vi "DAQ_PXI_NSCOPE.vi"(0 "Pre-Check Cut-Off (V)":dbl=0.5, 1 "Range Ch0 (A)":dbl=10.0, 2 "Range Ch1 (V)":dbl=10.0, 3 "Frequency (fp)":dbl format="%.10f", 4 "Sample Rate (fs)":dbl format="%#_10g", 5 "# Pre-Checks <1Hz":i32=1, 6 "# Pre-Checks >1Hz":i32=10, 7 "Oscilloscope":refnum<k15>, 8 "FGen Handle":refnum<k15>, 9 "Potentiostat":refnum<visa-resource-name>="Solartron1287", 10 "Auto/Manual \nSignal Averaging":bool, 11 "file path (dialog if empty)":path, 12 "Write Time Data":bool=TRUE, 14 "# Periods (Np)":i32, 16 "# Samples (Ns)":i32, 18 "Manual # Signal Avgs":i32, 20 "Frequency Run #":i32, 21 "Amplitude Run #":i32) -> (15 "Solartron Error":bool, 17 "Error code 1":dbl, 19 "Error code 2":dbl, 22 "Pre-Check Voltage":dbl[](graph), 23 "DAQ Error":errorcluster, 24 "Measurement Complete":bool, 25 "Cut-Off Exceeded":bool, 26 "Avg Data (FFT)":cluster{"f0":dbl, "df":dbl, "magnitude":dbl[]}[](graph), 27 "Avg Data":waveform(dbl)[](graph))   [LabVIEW 2018]
uses:
  <instrlib>/niScope/Controls/niScope trigger slope.ctl
  <instrlib>/niScope/Controls/niScope trigger source digital.ctl
  <instrlib>/niScope/Controls/niScope timestamp type.ctl
  <vilib>/Analysis/baseanly.llb/Mean (DBL).vi
  <instrlib>/niScope/Configure/Trigger/niScope Configure Trigger Digital.vi
  <instrlib>/niScope/Acquire/Fetch/niScope Multi Fetch WDT.vi
  <vilib>/measure/maspectr.llb/FFT Spectrum (Mag-Phase) for 1 Chan.vi
  <vilib>/Waveform/WDTOps.llb/WDT Get Waveform Time Array DBL.vi
  <vilib>/Utility/file.llb/Write To Spreadsheet File (DBL).vi
  <vilib>/measure/NI_MAPro.lvlib
  <vilib>/Analysis/NI_AALBase.lvlib
panel:
  in  "Tab Control 2":enum32{"Time", "Frequency", "Combined I & V"}(tab)
  out "Avg Current":waveform(dbl)(graph)
  out "Avg Voltage":waveform(dbl)(graph)
  out "Raw Current":waveform(dbl)(graph)
  out "Raw Voltage":waveform(dbl)(graph)
  out "Extracted Current":dbl[](graph)
  out "Extracted Voltage":dbl[](graph)
  out "Avg Voltage FFT":cluster{"f0":dbl, "df":dbl, "magnitude":dbl[]}(graph)
  out "Avg Current FFT":cluster{"f0":dbl, "df":dbl, "magnitude":dbl[]}(graph)
  out "Raw Current (FFT)":cluster{"f0":dbl, "df":dbl, "magnitude":dbl[]}(graph)={"f0"=0.0, "df"=0.5129974680086571, "magnitude"=[0.009736686034974913, 0.0068890118193715155, 2.474273316925892e-05, 1.6666181662903927e-05, 0.00018520497481361043, 0.0002020324625728159, 2.9796423917391588e-05, 6.0835799956176654e-05, 3.832061972696404e-05, 8.00163268760432e-05, 6.187686325990989e-05, 0.00010881345143237041, 7.405664232045423e-05, 0.00024529678937191185, 0.00018081723997787064, 0.00013674830034827767, 0.00011578668138923653, 8.132508891103869e-05, 8.436909603493343e-05, 4.3539255195424374e-05, 9.411278296038275e-05, 9.313339616697858e-05, 0.0001904916031194703, 7.18188449372633e-05, 9.515352739845026e-05, 5.8372027209711544e-05, 5.1629081344813335e-05, 0.0001051888984279757, 0.0001017511048336494, 0.00012806290765685684, 0.00023723970211607696, 0.0003284196771042644, 0.00016311109700680552, 7.052872379484058e-05, 6.441909845264623e-05, 8.963484915660137e-05, 4.660091676692494e-05, 1.1473371550415868e-05, 9.8723227863399e-05, 0.00018172145612905383, 0.00036925666576389734, 0.00020825496534972575, 0.00014413683504899518, 0.00011289417085277834, 0.00015953426281898876, 0.00017884377671758568, 8.647602637233157e-05, 3.0610648821725594e-05, 0.0003660063662156784, 0.0005702868602461952, 0.00021324756350599438, 0.00014543243135490178, 0.00014364891510409427, 0.0002982096066457441, 0.0002189892710822117, 7.654008130455015e-05, 9.377522933847826e-05, 0.00018913059395761627, 0.00013606168893038421, 9.838731433003454e-05, 8.098815429925746e-05, 6.508812680274274e-05, 9.860214326190474e-05, 1.1326564628447644e-05, 8.342745136118874e-05, 0.00011200339065280742, 0.00018218423703807567, 6.457659894070577e-05, 5.9605112794137545e-05, 2.0063007064420637e-05, 6.585541984966144e-05, 0.00013007463904747007, 0.00010747989177496173, 6.34156482784896e-05, 3.2140842110284324e-05, 8.656295230172939e-05, 7.554294012686232e-05, 2.9555901488047962e-05, 5.44336799610027e-05, 5.9179056867187395e-05, 3.177348946688188e-05, 0.0001589373764824556, 0.00020007344057657424, 0.00016532419934993018, 0.0002195032937442199, 0.00012792030895095305, 2.6877514530374027e-05, 5.175553268101543e-05, 9.242982765959301e-05, 0.00010891953547865583, 8.794904421914407e-05, 4.997279996143813e-05, 0.00010340449341237465, 0.00017928269490357894, 0.00011400343578560216, 5.16705631906662e-05, 3.995921618814623e-05, 8.877098180368605e-06, 0.00015421538895628968, 0.15339177843082097, 0.3079863886415542, 0.15456404384839195, 0.00012939967441387507, 5.376758334077757e-05, 0.00015723457526394858, 0.00011325594804700243, 0.00010475126580808048, 7.106805692341232e-05, 4.461115944250017e-05, 4.5035497990061865e-05, 0.00014599202683489022, 0.00019381744055934879, 0.00012660788832777155, 0.00010631495550691035, 5.8015657316982975e-05, 4.897213627895938e-05, 3.845893709285947e-05, 4.698686272509827e-05, 5.639004143367423e-05, 0.00013921113063345098, 0.00014851999400272212, 0.00012015584002173139, 2.2919384027760592e-05, 7.072686143507398e-05, 8.646597179868744e-05, 2.3574377975237496e-05, 7.834446303479069e-05, 0.00012318313764416266, 0.00011873834413899145, 7.099237231702384e-05, 2.7940946503255326e-05, 2.6690504994345562e-05, 8.092354678179886e-05, 0.0001481231603102316, 0.00012968992675136646, 3.454139667209186e-05, 6.526155774761239e-05, 9.300479469875524e-05, 3.0392342344455383e-05, 2.6396648157025413e-05, 3.867706349844679e-05, 4.275876334056742e-05, 8.387522147494939e-05, 8.388762532766892e-05, 5.251504295345165e-05, 4.161900465252819e-05, 0.00011192486472668473, 0.000114834446358765, 5.947076800455082e-05, 3.317368982212232e-05, 2.9931490166628703e-05, 2.494336068282783e-05, 8.751156553829414e-05, 7.875126342066757e-05, 8.716511963950046e-05, 7.702867210387553e-05, 2.8050096914227305e-05, 7.303259959720835e-05, 0.00012900223836404033, 7.72471266661751e-05, 1.0825078154982671e-05, 3.588740189973794e-05, 3.412256892415188e-05, 3.374013425044886e-05, 8.078331083064204e-05, 5.692432646868846e-05, 3.3647503843830784e-05, 3.775988882787654e-05, 7.275279727320078e-05, 6.949533452311763e-05, 0.00011832191062124111, 5.60299537837104e-05, 6.523885016889611e-05, 2.414308383480744e-05, 8.488677777026249e-05, 8.059614949570702e-05, 0.00012765831871195473, 0.00015327769066343622, 9.982504766895197e-05, 8.067231055434007e-05, 7.562952469606737e-05, 5.2441647077166705e-05, 8.774798136367469e-05, 8.907484043261529e-05, 4.2626022386031635e-05, 6.629829475941237e-05, 6.007341862699493e-05, 0.00013978145341757655, 0.00011875778781368468, 8.445889428951863e-05, 8.16344140794912e-05, 0.00011652908390162308, 8.686981487586638e-05, 2.0202520212430367e-05, 5.6675358309870864e-05, 6.489700940556412e-05, 3.843468744669687e-05, 8.598439265372556e-05, 5.235259661977289e-05, 1.9505584006020315e-05, 5.4967258789082405e-05, 9.061164932565477e-05, 6.871078242479517e-05, 3.746490793119356e-05, 4.345746570583056e-06, 6.680794809066679e-05, 7.859384577137153e-05, 0.00013946180119439166, 0.00015026973409200598, 0.0001261811098802357, 6.638106768113638e-05, 6.714891135164813e-06, 7.285469936222993e-05, 0.00010025486142062482, 9.340855417396117e-05, 7.13680068546361e-05, 5.4394809470155064e-05, 6.610151345962155e-05, 8.101947070807833e-05, 9.65679717611424e-06, 7.494334931301856e-05, 8.716030749396753e-05, 8.759095241319934e-05, 7.009364663007274e-05, 0.00013040985988452123, 0.00011666946833255358, 8.541439449473249e-05, 7.349157135610967e-05, 5.071127389460994e-05, 9.03494173236385e-05, 0.00013630334293557154, 0.00016550562942030102, 0.00010244158226284989, 0.0005095114593234241, 0.0011040607462522514, 0.0005898797354733062, 8.460699629733707e-05, 6.63279576799476e-05, 7.276767016123001e-05, 9.678912553521579e-05, 0.00011103880036497153, 0.00010390481304795893, 6.723211967444307e-05, 3.3213886943143796e-05, 3.118368973763882e-05, 6.487871614283443e-05, 0.00011403356228342304, 9.961545112336088e-05, 6.042829517827356e-05, 0.0001060634480773622, 6.258637735352707e-05, 1.8767611570095386e-05, 2.2703655562442184e-05, 2.077155298560397e-05, 7.824021568470722e-05, 0.00011626638539470062, 0.00010789538386553134, 6.356140113315058e-05, 2.810239679935883e-05, 4.1775096500033935e-05, 4.607647467623639e-05, 4.235802568480506e-05, 9.104740577434752e-05, 0.00012622488464947946, 0.00011264774436154257, 8.91323109364551e-05, 9.376842798607555e-05, 8.964164862492874e-05, 5.236017496094289e-05, 1.2895474917283831e-05, 5.334432271514443e-05, 8.034685472454221e-05, 0.00011817447952261686, 0.0001016055140793108, 4.093545210834721e-05, 6.397618939265519e-05, 2.7474839384394434e-05, 8.763127512317331e-05, 6.707542704870795e-05, 2.8725232413302552e-05, 1.8017107811668353e-05, 3.8369194145327003e-05, 4.760212941143611e-05, 4.429291876691551e-05, 8.223134513211495e-05, 2.8310310472408665e-05, 4.4706761631630575e-05, 5.816965840260811e-05, 4.35017537930857e-05, 4.467012516597325e-05, 3.946515725898186e-05, 5.691639403547728e-05, 0.00012880744129362161, 9.772451248873228e-05, 3.3912165678514714e-05, 6.17894895191819e-05, 0.00012120627437940271, 0.0001201575820294547, 0.0001085905977033308, 0.00014559566484507596, 8.183886463368417e-05, 2.8953994913944367e-05, 9.657799789209553e-05, 0.00011258550821111594, 4.648209002050687e-05, 5.3750971725136403e-05, 3.245817318073464e-05, 4.9810938136752383e-05, 2.098530153804232e-05, 4.0986434519044244e-05, 1.62171770005793e-06, 6.1003960347686064e-05, 5.709747925701273e-05, 2.741664262162681e-05, 5.508192887786684e-05, 6.104251718802619e-05, 8.362732954581307e-05, 8.839931021231336e-05, 3.189452220701922e-05, 0.00011707895923538106, 0.0001445564751074485, 0.00011442583508313368, 8.905055501835022e-05, 0.00010030213185014967, 0.00010107518845689998, 6.256144387215386e-05, 6.06224533428129e-05, 4.071048604377221e-05, 3.604333177370025e-05, 3.4838493172495606e-05, 5.076623336050464e-05, 8.671222799159577e-05, 0.0001173064723575974, 0.0001490266478294354, 8.565813622945636e-05, 2.993245654881321e-05, 6.189121046054565e-05, 0.00015450812940270522, 0.00016439122756040005, 8.305348425077181e-05, 3.3650880921098876e-05, 5.1460026722577275e-05, 4.4080475501819375e-05, 1.9718762346583145e-05, 4.019192631583561e-05, 6.16280354471133e-05, 4.581307559653348e-05, 7.132076812468776e-05, 7.955624531825839e-05, 4.2853964794850806e-05, 3.6423011063342666e-05, 0.00014801122176452545, 0.00016093044889958237, 0.00010722240371521513, 0.00012350052965298084, 0.00013278815839330737, 0.00012124553101414693, 0.00010594975107531911, 0.00010402056646776084, 6.656200710418502e-05, 5.030208295263895e-05, 0.00013966255877616076, 9.284996782012796e-05, 3.143267597881713e-05, 4.440692708678103e-05, 4.919436029081937e-05, 6.714031688275334e-05, 6.907044421329024e-05, 8.978463840174823e-05, 0.00011999972926478699, 9.624308047471834e-05, 6.685931512769558e-05, 0.0001350330138229978, 7.231584621783556e-05, 0.000124191755290804, 0.00013602537193404393, 5.485262262014689e-05, 3.290832408203692e-05, 8.864254628663135e-05, 9.256403786052085e-05, 0.00010979341528415184, 9.671861892468958e-05, 6.402085877484647e-05, 6.254057256074885e-05, 7.391047540786645e-05, 0.0001375830250966501, 0.00013240222432106118, 7.504311886533425e-05, 4.728428632484807e-05, 4.219163594033604e-05, 4.3894564028540294e-05, 7.402932040891047e-05, 2.0692018869526677e-05, 9.58176723661448e-05, 0.00012859624045696066, 9.468245456234631e-05, 4.58987093578452e-05, 5.973134686001529e-05, 0.00015495789102867437, 0.00015225176035776775, 0.0001152660456485345, 4.3977865615331864e-05, 4.473302645723064e-05, 1.038476669389405e-05, 5.178689049318982e-05, 5.2317526868503626e-05, 7.731241913713737e-05, 4.76983333819832e-05, 5.8764068074275494e-05, 8.050069369254132e-05, 6.607874793802826e-05, 9.048851015371822e-05, 5.0457073148019415e-05, 5.7353792645631936e-05, 8.30515433947444e-05, 2.0042899991487215e-05, 6.113036598742393e-05, 1.946816512274226e-05, 0.00011694111993686107, 7.523172257108798e-05, 9.476294475960118e-05, 0.00013860243809227297, 5.750702760830358e-05, 3.449398233058162e-05, 2.0956641714305812e-05, 2.1504301397232258e-05, 2.7471314957223322e-05, 9.381956771213715e-05, 2.922399583610309e-05, 6.942601588233773e-05, 2.779566295309615e-05, 7.130318946635892e-05, 7.149886430032594e-05, 5.139993358555985e-05, 6.362965788886956e-05, 7.596950087307978e-05, 7.140824565915071e-05, 5.805928359111721e-05, 1.9495487430821023e-05, 4.358710065559153e-05, 9.296638765574948e-05, 5.266407431067206e-05, 7.07958794194355e-05, 8.291348410989419e-05, 6.84661064625638e-05, 7.36777681683598e-05, 8.460517719374566e-05, 5.706680481474532e-05, 5.345143266824526e-05, 4.847036735315841e-05, 2.8214153312565667e-05, 1.578981545533103e-06, 2.420611739278338e-05, 2.5751830567147358e-05, 8.551775498456529e-05, 8.40121859158837e-05, 0.00012635421296699418, 0.00013810496120021876, 9.654466187198543e-05, 7.264826703182078e-05, 8.86819458827062e-05, 3.739617614081658e-05, 2.1572774041456367e-05, 7.405230908668645e-05, 1.0634229827824527e-05, 4.863725308657675e-05, 2.5670242337372567e-05, 0.00030464009896232825, 0.0005215942494986065, 0.00023890089645853916, 5.956385733777223e-05, 3.343738832445387e-05, 7.82343282299264e-05, 7.76107611911919e-05, 3.5356303122637964e-05, 4.9904972391740515e-05, 7.820723201161031e-05, 1.9497081628196724e-06, 9.509232738427502e-05, 0.00012178960632160106, 8.708742033778925e-05, 4.6179588317505504e-05, 7.220912813633792e-05, 9.487815934803574e-05, 0.00013352886336675827, 0.00012944982536255647, 7.347165394621793e-05, 7.378572299473907e-05, 6.868232364642505e-05, 3.152914516619926e-05, 5.081113626186942e-05, 6.410974432711068e-05, 3.3844879974463526e-05, 2.1381637242241187e-05, 8.802911475046838e-05, 7.795492847295635e-05, 4.6401157514948504e-05, 8.296667953849861e-05, 6.300370490185061e-05, 3.9815079382668113e-05, 2.0554859209610595e-05, 2.668634819337046e-05, 3.0594895727724854e-05, 0.00010101228045521858, 7.452174078973984e-05, 7.301396351874438e-05, 5.0361131639115245e-05, 0.00010223885869558667, 7.870120595035575e-05, 3.4195268663717826e-05, 6.993431704109734e-05, 6.784840022167438e-05, 7.877167330164065e-05, 0.00010830351213846695, 4.310256473271412e-05, 5.088589229695461e-05, 3.8889831648106724e-05, 5.313555049798199e-05, 8.937071224748178e-05, 6.366417181000868e-05, 2.6834658547450883e-05, 4.930678366103415e-05, 4.433978719036367e-05, 5.422573682040931e-05, 6.938892015234025e-05, 3.797906339025046e-05, 1.4884417747442926e-05, 2.6187539592185155e-05, 2.2060509314554238e-05, 3.950479262181867e-05, 8.748630975935549e-05, 7.297456341840467e-05, 4.443715821877729e-05, 3.8906913627877566e-05, 8.588731009112597e-05, 0.00011488789170993853, 0.00010509325331548041, 5.8581152791150975e-05, 3.1375583251849565e-05, 0.0001124421149809163, 0.00011647014056875088, 3.698400686923493e-05, 3.932625646119888e-05, 8.815761881254883e-05, 4.9728221439491366e-05, 2.7597546682014243e-05, 4.932919207824848e-05, 6.400269716373524e-05, 4.1488000643268364e-05, 0.00012369789792028514, 8.184587484456742e-05, 2.2257814390089976e-05, 5.836101829959298e-05, 6.053919224290029e-05, 2.160986785547073e-05, 6.684044861256318e-05, 9.936874323743204e-05, 0.00013202011193461338, 0.00014768737320262708, 3.08425032062915e-05, 5.4153579994495385e-05, 1.889707505957545e-05, 4.0234129979895406e-05, 6.708010932003336e-05, 0.0001036576812750676, 1.887118837445916e-05, 4.5727314718384076e-05, 2.1801911253719777e-05, 2.1702554484258357e-05, 6.0057071466645535e-06, 7.726596523730339e-05, 0.00012288780656647378, 0.00010748058602949488, 0.00010927847110088178, 7.566017112974956e-05, 5.434481261853587e-05, 5.2259295868476605e-05, 0.00012236560018837668, 0.00011967397383267307, 0.00013137412972701417, 6.821904344461343e-05, 9.901613754571401e-05, 7.325235838812019e-05, 5.5230935393848205e-05, 0.00011865463490682233, 9.780742744772071e-05, 9.944388518323193e-05, 1.5621224943444166e-05, 5.6737278656342645e-05, 1.130476823449511e-05, 7.567191277607406e-05, 5.661733529281561e-05, 3.697517880681608e-05, 4.7259278007570486e-05, 2.1150705524070954e-05, 5.0408740133679675e-05, 9.742431811289342e-05, 6.043880371443366e-05, 5.4216773363560614e-05, 9.741628508723267e-05, 5.26631847148604e-05, 7.404145166278438e-05, 4.854089759956882e-05, 4.084591046226174e-05, 9.647779744532907e-05, 0.0002086788569078152, 0.0002816364008376485, 0.00012688492199090115, 7.65944894577067e-06, 3.6243190873773735e-05, 5.6219245442062214e-05, 6.482549957968103e-05, 5.952284780214933e-05, 0.00011776869267202251, 6.297764469578426e-05, 5.049489135205378e-05, 8.957388997282253e-05, 0.00012178069093347264, 0.00012994116700553327, 8.65462049613954e-05, 0.00010317293890996919, 8.780074942067528e-05, 3.7070894249722783e-05, 6.063838953162865e-05, 3.8711820408366346e-05, 7.365089012689186e-05, 0.00012167617703242242, 7.463535257145054e-05, 6.744796912337132e-05, 0.00012547238865821364, 7.420593415086781e-05, 1.3265146026887127e-05, 3.778281860584183e-05, 9.263580341779995e-05, 0.00011127482344407767, 5.448048363772164e-05, 9.4835312810856e-05, 0.0001061324583135292, 5.304174882175788e-05, 1.3655344959992683e-05, 7.534164169987058e-05, 0.0001097624891031946, 9.892567197808427e-05, 6.440290146490046e-05, 3.359465023355497e-05, 3.336489617351486e-05, 3.7347271909427096e-05, 1.114351713994515e-05, 1.3280011245846888e-05, 5.7653718644720045e-05, 0.00011376458333905705, 0.00013508519802240597, 0.00015007176037114362, 0.00012605227107725882, 0.00013846080349423415, 9.672450350812372e-05, 8.162393719336778e-05, 8.439681307267638e-05, 4.9305198547823205e-05, 4.916116025882728e-05, 3.679531560280544e-05, 3.381976564598855e-05, 6.800270558935843e-05, 3.883778182696598e-05, 6.619844159553289e-05, 3.61327174348247e-05, 9.899844608661397e-05, 9.641573314022669e-05, 0.00013029877426087654, 9.792622843360607e-05, 9.612773349342937e-06, 0.00010595093656469532, 0.0001062997603506521, 2.0638875230808467e-05, 6.528101510225899e-05, 9.141616308402741e-05, 0.00013000443512000792, 7.352777259967708e-05, 5.8283219779554e-05, 0.00013024724166868325, 7.676376072054004e-05, 4.4004255152320334e-05, 7.377748909308422e-05, 7.282799041503763e-05, 0.00011915254383764491, 0.00013084000234690014, 0.00010875779185399029, 1.8182737075271514e-05, 8.146683382542437e-05, 5.285316001041333e-05, 5.444536450416586e-05, 8.893395805738149e-05, 8.791719908479843e-05, 1.0596102287905125e-05, 5.5376573877938076e-05, 4.445148438988052e-05, 1.3065696408997875e-05, 4.905682607771033e-05, 5.495912985831932e-05, 6.671294454519575e-05, 0.00017614598241608352, 0.00024936876686896593, 0.00023075568028057064, 8.174648183910437e-05, 0.00012832008811656343, 0.00017120686073142003, 8.001791157475066e-05, 5.5262032197503914e-05, 0.00011954837203916514, 0.00014131364608077743, 7.494576556768572e-05, 1.9258150894335585e-05, 2.4689531873113616e-05, 4.100126605219083e-05, 5.5407081228469744e-05, 3.342161763723121e-05, 7.411251564025284e-05, 0.00010266237821433993, 4.365990864847796e-05, 0.00013273480744348552, 0.00010514576472763523, 1.6401965324536744e-05, 3.330547168281681e-05, 5.4876593797890525e-05, 4.1872340037192876e-05, 5.316806803893302e-05, 9.527289462861894e-05, 0.00011932291188269206, 7.07878166763032e-05, 6.140773852560813e-05, 0.00010575849170671164, 3.55693637829357e-05, 0.0001702915367426079, 0.00013198694888416797, 8.719038762157511e-05, 5.8237878386127945e-05, 3.594218835046773e-05, 7.429942605156042e-05, 0.00010349793151274568, 8.551902937563557e-05, 4.514467811784512e-05, 0.00012067802796381594, 7.57907618242714e-05, 7.823011660290687e-05, 0.00010940165977071781, 8.514772365347824e-05, 7.064968219620165e-05, 4.6265666573087246e-05, 3.100548241734962e-05, 4.3039765824007554e-05, 3.557281979382924e-05, 6.790993980024899e-05, 6.976697801962028e-05, 7.416516495684897e-05, 3.066179330092311e-05, 4.82093392389968e-05, 5.6035858550855465e-05, 0.00014238507566795853, 0.00012837569468342303, 4.7836322519587243e-05, 4.090600853776808e-05, 3.8623802708545994e-05, 1.0920860638683462e-05, 4.484421167162386e-05, 4.044967384052889e-05, 5.262324800317312e-05, 6.444345034878788e-05, 0.00012934770560551456, 0.00012532575141136143, 5.113134222634911e-05, 2.5216446871126786e-05, 7.096580006339864e-05, 9.079397535182139e-05, 2.9688993541135436e-05, 0.00012210308543205396, 0.00015444737990201693, 3.5927516997820995e-05, 9.783678721341039e-05, 8.403266144624943e-05, 2.282976613095964e-05, 2.4239904920084537e-05, 2.9592721920004422e-05, 7.465726173416601e-05, 8.068614973947232e-05, 7.093577123693782e-05, 0.00010412829958033035, 9.732216827165277e-05, 5.930575290373523e-05, 0.00011457345386857833, 2.8518905900681316e-05, 2.1936126073443543e-05, 2.8825167081171048e-05, 5.93289117939227e-05, 0.00010209438069501936, 0.0001162370205311875, 4.987420116396371e-05, 0.00011979834313332878, 0.00014711114330424782, 0.000122187845606995, 7.252318340228763e-05, 7.570534940278734e-05, 6.08384890721689e-05, 2.7986426863347572e-05, 4.722924819400313e-05, 5.854346874367302e-05, 9.255160605113158e-05, 0.00010164143314471596, 5.5626096348192946e-05, 2.4038674553347115e-05, 2.8302447295059293e-05, 4.733825719690651e-05, 0.0001127536977895883, 0.00014250397904411297, 0.00010386681879613563, 3.83053126598355e-05, 6.338939647529567e-05, 6.188875910509229e-05, 0.0001299309427061446, 0.0001387621466422242, 0.00010658429185122108, 9.21768261458646e-05, 9.511093033946011e-05, 0.00012935323400315842, 0.00010108674281125153, 3.695887288357596e-05, 2.3353610099248402e-05, 7.621964101659557e-05, 0.0001320341958591496, 0.00010944232875996149, 0.00013403921594062809, 8.008460821005282e-05, 6.328943108465424e-05, 5.2672991184966514e-05, 9.285796299526138e-05, 0.00014128959312560127, 6.506509471810883e-05, 4.2120328583756805e-05, 4.019775672648957e-05, 8.073242584600459e-05, 7.85784793203739e-05, 2.4112589175674725e-05, 4.787838631254602e-05, 1.8493998234257306e-05, 2.102294091265015e-05, 8.585783935453163e-05, 0.00011711203744278809, 0.0001380507068111013, 0.00010905344470843212, 7.628261895217422e-05, 4.667606884598736e-05, 9.718331171415582e-05, 0.00010828985400035679, 4.01628869688618e-05, 9.894226174474573e-05, 4.020560493018181e-05, 1.1689809911468847e-05, 3.0255734845274146e-05, 5.134463794730575e-05, 0.00010907399556691874, 7.973482277266835e-05, 6.722145293054134e-05, 0.0001053169606419433, 4.672146823500862e-05, 5.0539303928871415e-05, 4.8331253016411217e-05, 9.746834923478947e-05, 7.698571800967268e-05, 4.125281773340443e-05, 7.033043184967756e-05, 8.726104290370659e-05, 9.99268254883657e-05, 5.675302645371635e-05, 9.958379275426882e-05, 0.00016827405894896197, 0.00013964759385613767, 8.95549592619375e-05, 7.897571682700118e-05, 6.128746920052035e-05, 6.632258195704656e-05, 6.968881001225131e-05, 7.660022716412855e-05, 0.00010285727745289522, 8.364884815307242e-05, 4.967183102917859e-05, 7.873564670159473e-05, 2.8431073344225065e-05, 0.00011887695069708306, 0.0001386807050420087, 7.845114993305462e-05, 7.501684244765425e-05, 7.655588025221887e-05, 3.417251832136325e-05, 2.465933953351524e-05, 7.675505197378193e-05, 8.774302621367597e-05, 6.954442321748203e-05, 3.4345394042422326e-05, 6.91084206103343e-05, 8.603371623311356e-05, 2.08788859685803e-05, 0.00011747715884471567, 0.0001590319637305697, 9.16542858579216e-05, 4.135831001374284e-05, 4.93906784129331e-05, 6.63191370159788e-05, 7.626841953447927e-05, 5.761164745744449e-05, 5.307108376029597e-05, 5.8823539706247943e-05, 3.441272657484893e-05, 1.297825006753756e-05, 5.789994837285246e-05, 0.00010732593218108915, 7.135371759510655e-06, 0.00010682252977078337, 4.826518290433291e-05, 0.00012217170255594633, 8.898579102329243e-05, 9.04571670529567e-05, 0.000137906168767138, 7.01221516471587e-05, 5.555009661169892e-05, 5.562932049465801e-05, 3.6708423205372413e-05, 3.1710904103314065e-05, 6.77313338328506e-05, 0.00010935049915680121, 7.406214816050558e-05, 3.830638640461101e-06, 8.141981164838396e-05, 9.674105614198826e-05, 3.852252315554934e-06, 5.8673701338300754e-05, 9.560119732944193e-06, 1.2468650315511109e-05, 2.2580391310606328e-05, 8.4699281855885e-05, 3.616555630609264e-05, 6.0242524367222254e-05, 3.7887000817292114e-05, 9.723355489476523e-06, 0.00011497438687740393, 9.887099374371441e-05, 4.968501196928022e-05, 5.030401191366171e-05, 7.697130041308423e-05, 7.913195957848586e-05, 0.0001089804841219723, 0.0001331567938024021, 6.716304425071966e-05, 0.00011416210294702766, 0.00011636997103350444, 5.182024596318364e-05, 5.138795450705537e-05, 2.7076177830046352e-05, 8.565879568166872e-05, 6.0732640651598016e-05, 5.063408706388943e-05, 4.433718014835687e-05, 5.0204412665408934e-05, 4.787562591066475e-05, 6.4906011338989086e-06, 0.00011416805100848756, 0.0001246392522080917, 2.4470860730452252e-05, 6.292790176716217e-05, 5.607839392326423e-05, 6.919123072865869e-06, 4.760260501554702e-05, 6.355851848049534e-05, 5.3553551803857856e-05, 0.00012622125762591353, 7.599771217613932e-05, 5.6808019470107833e-05, 7.239290855550899e-05, 5.849455279273172e-05, 7.934472020911803e-05, 0.00010550105017455192, 5.4620645915706855e-05, 6.86758349387712e-05, 2.8368495390775327e-05, 6.569041242177681e-05, 6.68619356519367e-05, 4.5391570998620266e-05, 2.6026697622941814e-05, 2.9029515552678967e-05, 2.593718695821507e-05, 4.2954470354591866e-05, 3.09612681132032e-05, 4.391713215084827e-05, 4.669939343076136e-05, 5.141138152043193e-05, 3.835081174329836e-05, 1.6017096517240038e-05, 5.39049349126851e-05, 6.465699944047969e-05, 5.210794840750768e-05, 7.468255806654975e-05, 2.3789285868340063e-05, 0.0001184437626939303, 3.443352849048159e-05, 3.578786209871268e-05, 3.547327402633728e-05, 4.3737768060141656e-05, 5.745004643225023e-05, 2.3542254816754582e-06, 5.655420587348942e-05, 8.314204844720425e-05, 5.9657472749715766e-05, 3.664022410474088e-05, 0.0001148120544600091, 8.939767481534439e-05, 5.023100718699245e-05, 0.00010813732941925436, 8.494862157990408e-05, 8.733457168212002e-05, 5.955545570006324e-05, 1.9924278172100827e-05, 7.207335653920181e-05, 5.252879433140767e-05, 5.045635532042773e-05, 8.951432528177735e-05, 1.8460637180872944e-05, 9.222590951048993e-05, 6.954340686450249e-05, 2.1040582881605123e-05, 4.788370106216473e-05, 3.2169955738500416e-05, 9.980405334476289e-05, 4.045951328994319e-05, 8.994470620340262e-05, 0.0001217962045519954, 4.580705365775434e-05, 5.168848122163649e-05, 8.882206357593652e-05, 0.00010217459843757783, 8.487861710537117e-05, 0.00010100790099996582, 0.00013651019546828905, 0.00014885935698358524, 0.00013435973668555912, 0.00012681820332396097, 7.788683493468936e-05, 4.719188328881677e-05, 7.42134396930508e-05, 9.654159845424399e-05, 9.792391262325924e-05, 4.938300479744665e-05, 5.827843733149042e-05, 3.239784247671153e-05, 0.0001651178247974607, 0.00019193477971505418, 0.00021368424717870275, 0.00013185083154650012, 1.9521067740372554e-05, 0.00011647477793580137, 0.00013219511677418103, 4.7091913331635426e-05, 5.592704760289938e-05, 9.229918757236661e-05, 4.045862513745276e-05, 6.129907877749199e-05, 2.5994795835360393e-05, 6.986717008082854e-05, 1.3402979680291646e-05, 3.537934738868749e-05, 0.00010874591203650715, 7.564219759013805e-05, 5.9896174545815454e-05, 6.805640161783559e-05, 2.8185354120430034e-05, 4.027054696526677e-05, 3.4811618518767625e-05, 6.534176687240436e-05, 7.250849374147664e-05, 0.0001555073809743529, 0.0001245114364012905, 8.546002362091024e-05, 0.00012460821285001743, 0.00017201139751436514, 0.00017199255975052118, 7.565527982564014e-05, 7.23877719835643e-05, 0.0001542426407384879, 0.00015573276483068016, 8.94266924162458e-05, 9.082483391685248e-05, 0.00011400344675558218, 1.3158318706717286e-05, 0.00010189119555680978, 6.094548486393501e-05, 6.995790757341798e-05, 9.142914634282154e-05, 5.6710074212175546e-05, 3.5615630698560994e-05, 8.896155900995747e-05, 3.1236595793982005e-05, 7.69757153335617e-05, 6.374685234551762e-05, 3.1149793320846253e-05, 1.4030337410335409e-05, 4.499972918124282e-05, 8.018904215107677e-05, 8.013939385620256e-05, 0.00012356212307987666, 9.661533785137773e-05, 4.400898053700234e-05, 2.1524092202036146e-05, 2.0888608040520335e-05, 2.8210970848255015e-05, 3.52042915785868e-05, 6.470210743827551e-05, 0.00014491759767358054, 0.0001229716959917464, 0.00013064677818916198, 6.944931919737882e-05, 6.2943643625256775e-06, 1.4023829852767115e-05, 2.5367320673109177e-05, 8.793344480173676e-05, 0.00011023073751234149, 8.601579486915851e-05, 7.719475877412213e-05, 9.105332233657286e-05, 6.02837981894214e-05, 2.5261728381191385e-05, 6.323309482102024e-05, 6.600251568271427e-05, 5.469087080920579e-05, 7.1362407823795e-05, 5.603973578987791e-05, 3.0711932252435064e-05, 4.2333118627721086e-05, 6.0543398631587896e-05, 2.503952953985616e-05, 0.00011581570336427287, 9.889701049604456e-05, 4.987980933973253e-05, 1.704673406180222e-05, 2.138043084768542e-05, 3.931841269478685e-05, 4.912854297038053e-05, 6.80522650667397e-05, 0.00011118575599479467, 5.69795060165624e-05, 9.383317094273614e-05, 6.50242539850638e-05, 9.67760844771563e-05, 4.182786376653853e-05, 4.3092827333801965e-05, 6.755793174594356e-06, 8.607607029774266e-06, 5.557776983427308e-05, 0.00010287596735457048, 0.0001159846897373211, 0.00018085811623493077, 0.00011734192003755868, 4.4905187830937135e-05, 6.408202711170145e-05, 0.00011187451004898436, 8.860668065633452e-05, 6.736671323606547e-05, 0.00011029639894262655, 5.3954791360589355e-05, 2.1241782644523725e-05, 1.0381124286379151e-05, 1.9372417418389157e-05, 2.6270507639902297e-05, 7.417575863277701e-05, 0.00016131914111586798, 2.2509271824866267e-05, 0.0001413959480718631, 0.00010788342553119171, 4.897915597212374e-05, 1.6768738982695494e-05, 5.682551383141501e-05, 3.2469246296295584e-05, 2.730718209966202e-05, 4.670975090435728e-05, 5.651485595244382e-05, 6.0553934793525154e-05, 5.209766983284627e-05, 4.116487485013445e-05, 4.022808166339871e-05, 7.598291292934882e-05, 5.346343243672562e-05, 6.210995491712195e-05, 8.230440771696741e-05, 0.00011581622548749921, 9.708832763604018e-05, 9.054211988620269e-05, 0.00010019746047959684, 0.0001000241585182197, 6.0483782737894455e-05, 4.717148726819008e-05, 0.00012416044405786798, 8.501296957991087e-05, 0.00010428848761483963, 0.00015888375923021512, 0.0001592056106987543, 9.219535559178928e-05, 7.262528760170768e-05, 7.117679784352188e-05, 4.27481280885166e-05, 6.064685960260453e-05, 1.1332587355937405e-05, 4.294126765271278e-05, 8.81359432677043e-05, 8.550299799381882e-05, 4.311227336669742e-05, 4.755027850677535e-05, 8.569015674632077e-05, 8.179995549832732e-05, 4.6883847476086586e-05, 4.9330273505091774e-05, 3.037769204953404e-05, 6.871609151127021e-05, 8.536526739843539e-05, 5.396248805577197e-05, 5.1620967281484684e-05, 5.1456862946303014e-05, 4.2652433115283795e-05, 0.0001080544904055672, 7.703919699348674e-05, 1.8221547918931794e-05, 3.0232382465296556e-05, 4.589931518736616e-05, 2.0900031542733726e-05, 6.863004927081564e-05, 0.00017374355797650036, 0.00011652343705188037, 2.1738060754054874e-05, 1.9836622911033635e-05, 2.823543649235006e-05, 7.953501985976011e-05, 7.834497530094624e-05, 0.00012235951285942208, 0.00012843151242013657, 0.00010511024217702175, 5.259322078153344e-05, 4.6286420328241075e-05, 2.88600300106447e-05, 5.891397424689143e-05, 4.8123551507112466e-05, 4.446391483076436e-05, 7.081734855694279e-05, 7.447209064193473e-05, 8.295991090554601e-05, 5.618781898660279e-05, 5.1354457129577643e-05, 9.083447212969017e-05, 6.154890931838974e-05, 4.953098172389299e-05, 4.206468390191532e-05, 9.52545153360766e-05, 0.00013556846728926745, 3.4868557980771985e-05, 8.164743314263412e-05, 5.151548866859173e-05, 9.11155510513629e-05, 6.17406430549882e-05, 8.601213925646853e-05, 0.00013015036634028248, 8.405223491410596e-05, 5.749898498164484e-05, 2.0994360829929272e-05, 5.927473271504225e-05, 9.591805523980466e-05, 3.813789829572376e-05, 0.0001014084740597618, 9.996128195684985e-05, 4.729133626555237e-05, 1.6378855787677934e-05, 6.426790632722436e-05, 8.184663616184083e-05, 0.00010839702687940286, 6.690871343470749e-05, 8.253965986958716e-05, 0.0001246973784528823, 8.747217544938053e-05, 9.636425937037807e-05, 0.00011726190701598256, 3.440639779503234e-05, 0.00013540818941792614, 0.00017054719457821284, 1.5505362529250287e-05, 7.177217805375034e-05, 1.9742007531421337e-05, 5.851138717366113e-05, 0.00013604238423252905, 0.00013683083284163713, 0.00011968899493300909, 7.109103331838126e-05, 5.8856495019582197e-05, 2.796572793047781e-05, 3.085363139621229e-05, 2.81575275507043e-05, 1.388706387496167e-05, 3.051256648284573e-05, 1.3945480049738817e-05, 4.181087351330221e-05, 8.072378899496761e-06, 7.990931711066315e-05, 8.664966942695761e-05, 5.292257837319129e-05, 6.428003834638072e-05, 3.686312542674316e-05, 0.00013453789367506033, 8.391026559501183e-05, 5.7429477640186194e-05, 1.3137523578609169e-05, 2.2945408248717663e-05, 1.7444109217037267e-05, 6.31685176943064e-05, 8.405972046680426e-05, 7.568038590893096e-05, 0.00014789623774038056, 0.00016345173454802633, 5.9143659260903816e-05, 2.355271871607092e-05, 6.50207254924217e-05, 0.0001277433320307822, 8.46824109161955e-06, 0.00010893869330525662, 5.365068338167295e-05, 3.332186339806504e-05, 6.633498511402389e-05, 7.032302427769354e-05, 6.293605649415344e-05, 3.2779160431872945e-05, 5.003840367373862e-05, 8.148365724422335e-05, 9.882527171233261e-05, 5.636912199020016e-05, 3.085180993351448e-05, 5.5244173718013026e-05, 5.502019666713831e-05, 6.505051365827459e-05, 3.9850111141789775e-06, 4.215695342839298e-05, 0.0001060044870478287, 0.0001352374815170716, 1.8998937715323976e-05, 3.5829797254728434e-05, 1.5033253868029578e-05, 5.246643580676588e-05, 0.0001030086140400812, 0.00011147577184680306, 3.642072107283331e-05, 5.726992849962852e-05, 0.0001398177087907839, 0.00014630856414124288, 9.414119181597995e-05, 6.359209645089427e-05, 7.799573345324339e-05, 3.5768659908926674e-06, 0.0001067908834390345, 7.909116601084773e-05, 3.9212939120793605e-05, 6.425301635572063e-05, 7.434819100468811e-05, 3.665951504513878e-05, 1.756992138592397e-05, 5.3833829068806206e-05, 4.4400561838383185e-05, 3.4854072806900566e-05, 5.293535362958484e-05, 2.8980961291710262e-05, 1.0649318805572046e-05, 2.7035756456528955e-05, 3.802596766763527e-05, 7.042548390122817e-05, 6.447321862377597e-05, 1.1445102541184316e-05, 2.4383184836101662e-05, 7.340943785201234e-05, 0.00011455829980455332, 0.00012022826874577315, 0.0001596791046387413, 0.00018775298406475166, 8.420089831255512e-05, 5.0067400228989605e-05, 1.1083266293860374e-05, 1.5552020242010087e-05, 4.653347750589265e-05, 2.3989411178119632e-05, 5.477170338134162e-05, 0.00010014371088002869, 2.2984353404798304e-05, 9.011054525341325e-05, 5.212777210184286e-05, 0.0001355937134226667, 0.00011919918769140552, 8.130366658569784e-05, 3.446692101220835e-05, 0.0001003563947378734, 6.440729547262126e-05, 6.287091225760104e-05, 5.347093032937117e-05, 7.680346774228692e-05, 5.5818744438868304e-05, 3.100357683282677e-05, 1.7242588977592983e-05, 8.135483951968637e-05, 0.0001209829936469434, 0.00011688688534437231, 4.912419526124349e-05, 8.894485008394771e-05, 9.799258821855075e-05, 0.00010807762257419386, 8.729454346275591e-05, 0.00010412181780226692, 6.189699862858598e-05, 3.0235209470920387e-05, 8.253775365930433e-05, 4.1023198533235374e-05, 0.00010472636344886955, 1.0632625210507553e-05, 2.3896957233777144e-05, 3.751791069351541e-05, 8.64452329271966e-05, 0.00010036903007620458, 6.507355385604517e-05, 9.199087509833584e-05, 5.608081582758995e-05, 0.00013121936180527838, 0.000156502862358784, 7.045833505913383e-05, 9.069439608758245e-05, 6.852928326556257e-05, 4.9282801720256094e-05, 6.93913868193009e-05, 4.165715971751554e-05, 0.00012171177514178709, 0.00010146704790968594, 4.906905315422634e-05, 7.965660455216568e-05, 4.906488314702306e-05, 1.024176325587832e-05, 8.399182685138372e-05, 0.00012579142019898774, 4.0100563107338616e-05, 4.9324933631228444e-05, 4.1383990898995025e-05, 7.396270274223919e-05, 8.970708234999438e-05, 8.816364734969336e-05, 0.00012082801087254325, 3.770697363815215e-05, 0.00011826232398438905, 7.229135950909975e-05, 5.336690781724693e-05, 8.354963822375454e-05, 2.3339348912803985e-05, 6.469020497655987e-05, 5.064130096908539e-05, 5.603422529971775e-05, 3.753546116241926e-05, 8.346080175677801e-05, 5.105828421636441e-05, 1.3772559594746388e-05, 1.0500419357342959e-05, 5.836181501549193e-05, 4.429666557845677e-05, 8.463920082676785e-05, 4.084429208069381e-05, 6.148446727108448e-05, 5.829324934446184e-05, 2.9059534594374283e-05, 1.8200181449152194e-05, 2.9013298749062535e-05, 2.1157903229715753e-05, 2.4909756636307545e-05, 5.9396824235009846e-05, 3.4597750875064926e-05, 7.01531323921953e-05, 2.6269865067543734e-05, 0.0001097039032900283, 0.00013097819539911948, 2.637949077043636e-05, 8.136621225148429e-05, 0.00013321592706127047, 9.881237436093312e-05, 3.794107452099959e-05, 1.5434123253124915e-05, 2.071705668804858e-05, 7.854149504225196e-05, 0.00012610977781006094, 0.00010278930531210562, 3.381769885525304e-05, 6.170667723261171e-05, 8.50039144171586e-05, 5.629646286721564e-05, 2.0058513383908546e-05, 5.74526730098044e-05, 7.40415694974769e-05, 7.964952619522259e-05, 4.727187953772571e-05, 9.24774297060932e-05, 0.00010079250907767682, 4.796723482055833e-05, 5.939045811756754e-05, 4.561099444147611e-05, 1.5147435314366943e-05, 1.9479009832401714e-06, 2.5012258712425605e-05, 6.448265791257708e-05, 2.8908738185949957e-05, 2.4829602182734974e-05, 4.209162414483849e-05, 6.622051561880598e-05, 0.00012809633440081158, 0.0001333174764336477, 0.00011519633516021489, 9.199882850616418e-05, 6.718308466116146e-05, 6.619477358073931e-05, 6.24549041101175e-05, 4.6646997281971245e-05, 7.606535665758584e-05, 6.382149608841462e-05, 6.58395326089848e-05, 6.913607587165692e-05, 0.00010314576204833388, 6.392279484441933e-05, 4.658913398904283e-05, 8.619223296222482e-05, 5.344023077991428e-05, 4.1994875998149234e-05, 6.564912168031801e-05, 9.460334353547627e-05, 0.00013307337593759753, 6.070480226900139e-05, 7.42568699635834e-05, 0.0001236092254652738, 5.215927365465155e-05, 5.0805588554635514e-05, 7.596752636148844e-05, 9.597288501832841e-05, 0.00010514543486867016, 0.00010273117411332805, 9.081727998292661e-05, 0.00011445861346242126, 0.00014551786276948577, 0.00015543241010492734, 0.00012032211273871897, 4.055340699527514e-05, 3.39441680160164e-05, 4.021611356129771e-05, 4.846979042047685e-05, 3.528139560736017e-05, 4.4463000731659834e-05, 3.9053083117581076e-05, 3.929185960436038e-05, 4.9628172454793196e-05, 8.204330450857583e-05, 8.944168434142099e-05, 8.691479967161323e-05, 8.082871232078013e-05, 6.0342343549756324e-05, 8.300521466494471e-05, 0.00010945627047477012, 9.114528465499299e-05, 5.9059658886007045e-05, 6.0394959108398155e-05, 8.619000713293784e-05, 9.170073834004933e-05, 7.875930605328551e-05, 0.00010090424100415313, 0.00015638193963645323, 0.00011061037477880064, 6.005192527925918e-05, 7.724630895477524e-05, 3.816941691693574e-05, 2.6777760138001573e-05, 0.00010799217973717106, 7.045983312977735e-05, 1.474584140927438e-05, 3.558795958464629e-05, 4.585423393501645e-05, 8.946001994944166e-05, 0.00011793371738616543, 6.730637563697642e-05, 8.98489806083701e-05, 5.822885149476587e-05, 3.369922165457592e-05, 4.261508552772883e-05, 2.6887192741679545e-05, 4.162386740411925e-05, 3.1168793876430404e-05, 4.597046069679254e-05, 8.7526464824867e-05, 3.6260599806371185e-05, 5.791658915600766e-05, 7.411321117559258e-05, 4.2052907662823005e-05, 5.7062035965089634e-05, 4.363158792611486e-05, 4.7743147444775106e-05, 7.859794288594684e-05, 9.072642886164255e-05, 2.1560854265676325e-05, 5.8735820431875444e-05, 2.5294183114247654e-05, 4.233862839288128e-05, 8.704160734418863e-06, 5.2538890400654945e-05, 8.49857203394752e-05, 4.810969533744059e-05, 4.9423212274192674e-05, 3.301520285289062e-05, 6.20302638228876e-05, 7.322516604443156e-05, 9.317763015494104e-05, 9.109620922760536e-05, 0.00010657134796681009, 7.391588316019145e-05, 1.9653780456160304e-05, 3.687561019767643e-05, 4.50330316455404e-06, 1.4563329932735234e-05, 3.0650720038187365e-05, 0.00011079294905594076, 0.0001231273201769807, 6.0745317595897405e-05, 2.3699432971041623e-05, 1.3163253099269776e-05, 5.200102277736974e-05, 7.166673622716148e-05, 0.00012830849139746665, 0.00014130892061055554, 0.00011004736730139153, 4.758098466601198e-05, 5.7883017839213974e-05, 7.962505514529395e-05, 0.00011167688196843098, 8.794327247697075e-05, 5.8115367223872305e-05, 8.410039975832879e-05, 4.0058700780115186e-05, 6.251684310286954e-05, 0.00011712923299676973, 7.357651725203104e-05, 3.628640510431301e-05, 4.4028895529066666e-05, 6.114377962702075e-05, 9.41284664185419e-05, 8.601390481131111e-05, 7.33695228603279e-05, 0.00010790274521847701, 0.0001072553461176403, 8.942253898758542e-05, 0.00011975275694118204, 0.00016900049442072868, 8.540892650377948e-05, 6.0967074853158266e-05, 3.2900668283086414e-05, 1.761883934805866e-05, 5.791395249878611e-05, 5.8768022283183874e-05, 2.79830111804684e-05, 5.293574040172161e-05, 0.0001315510193344673, 0.0001622739539539606, 0.00010041366770384316, 6.63603960471822e-05, 0.00015747965777463717, 0.00012878560641644074, 7.869153531534173e-05, 3.8059014088214166e-05, 3.769973943621439e-05, 7.742207172954492e-05, 0.00013089412757797647, 8.437661109462401e-05, 2.3324296223741458e-05, 1.0167496017936478e-05, 0.00010029780300179535, 0.00019447555680888684, 0.0001527782270298898, 0.00011884030727830697, 5.937196384587504e-05, 0.00013592129860328509, 0.00011578123354831381, 0.00010345475306570938, 5.50937128004907e-05, 9.704712627245555e-05, 3.3365209177347525e-05, 8.060199359458466e-05, 4.184442707242719e-05, 8.585955431688323e-05, 7.650757949647257e-05, 5.680584546171406e-05, 0.00016185629537601492, 7.9092984220475e-05, 5.510455104733978e-05, 3.54845584077038e-05, 0.00013920058161741384, 0.00013609053638422638, 7.680861189928892e-05, 0.0001687562205747208, 0.00016790589073789464, 9.651391033038544e-05, 4.0192732198884345e-05, 5.247739913211994e-05, 6.164214632583672e-05, 7.233556313460258e-05, 7.176296142846236e-05, 4.236873382092799e-05, 0.00010869221049457684, 0.00012759577785999033, 0.000103702571841759, 6.643467053826662e-05, 3.2770035232537e-05, 4.354708821417443e-05, 5.2289175436611046e-05, 9.783907359228593e-05, 0.00013264098806386033, 8.313405463070077e-05, 5.5194735414876024e-05, 8.692503225526954e-05, 4.756966377211389e-05, 0.00010720466180253656, 6.461366833122605e-05, 4.960281294763827e-05, 7.468503932466735e-05, 3.3496010463612296e-05, 0.00012497113065379812, 0.0001254958924832997, 4.915772645707733e-05, 2.8337615844899863e-05, 5.82863371460653e-05, 9.012194071659063e-05, 0.00012114273428867728, 0.00012446216749867106, 7.496623231657783e-05, 3.696039349454734e-05, 6.761380910193125e-05, 6.254799161472947e-05, 5.462586762783539e-05, 7.329385023661201e-05, 3.313518407250426e-05, 3.6581737132193786e-05, 8.008808689889343e-05, 0.00010710284231672867, 9.328500981498076e-05, 7.555224082660728e-05, 8.323021885733338e-05, 9.279547204802665e-05, 4.0677583586153764e-05, 3.689102450196697e-05, 5.1998453638488155e-05, 6.145274772402466e-05, 9.128816741381892e-05, 6.875827187371332e-05, 9.615302090327267e-05, 0.00011036807115062813, 8.612226657475793e-05, 0.00013531844348037872, 9.843392695596008e-05, 8.622199428216747e-06, 3.8674689645983634e-05, 0.00010630527507886132, 0.00012041630062075119, 6.933143297839332e-05, 5.1904146311599e-05, 7.819505226254796e-05, 2.3294356731909875e-05, 6.22845797345801e-05, 0.00011022691477430783, 5.369604053324257e-05, 5.898245294918871e-05, 7.454244631822826e-05, 7.879306465760291e-05, 0.00011542112111976764, 0.0001255666044061713, 8.777834336422177e-05, 7.215906366287644e-05, 8.285237447945316e-05, 0.00010932001280425939, 0.00011326061020514665, 6.730354951374269e-05, 2.3854805480784416e-05, 3.797582434843099e-05, 0.0001101848432170691, 0.00010909093697863792, 6.820866957751802e-05, 8.58404818202965e-05, 0.0001050570690912771, 7.635888438372816e-05, 2.446602347200826e-05, 5.925245953939786e-05, 5.90862647528598e-05, 5.5661119425029424e-05, 0.00011881461542306238, 0.00013519793202337443, 0.00011144694287596077, 4.487289627654631e-05, 9.39290242668394e-05, 0.0001380918995603799, 0.0001069531367997449, 8.905171488202379e-05, 0.00011936452022966949, 7.075528466570713e-05, 2.92878886815566e-05, 2.1328485908689197e-05, 3.849758796543818e-05, 0.00012075768011660604, 9.658944496122205e-05, 6.398696789497448e-05, 7.320710824906959e-05, 0.00013613994300246026, 9.64148558082593e-05, 4.5229120110167584e-05, 2.994018137707028e-05, 6.48658210872562e-05, 3.009692244233363e-05, 7.491383375523833e-05, 0.0001241587403709238, 0.00010160327357273639, 6.590742095988142e-05, 9.54454814703235e-05, 0.00010831226900531533, 6.421739389598407e-05, 4.994064457500763e-05, 4.136241964313395e-05, 2.616766252396583e-05, 6.66113843813241e-05, 0.00012146425545895542, 0.00010781475109632398, 8.571814066931091e-05, 7.090162024602478e-05, 7.930127910888381e-05, 0.00012961206856157155, 0.00017301280661145287, 7.929453719704741e-05, 9.175365921236214e-06, 3.6644855141514325e-05, 8.31243724371274e-05, 3.4093471591698445e-05, 5.001848398306565e-05, 6.556519425202842e-05, 9.746933013597654e-05, 8.924941232941476e-05, 0.00010870735455352234, 0.00012357968174474653, 0.00011293720755676026, 9.71181336564903e-05, 5.8767772763200484e-05, 2.2683607689607598e-05, 6.500658930637206e-05, 3.237270335970912e-05, 3.03516967301175e-05, 4.1257070322620795e-05, 2.0714862662684896e-05, 5.579677963314373e-05, 0.00011957101263186114, 3.815646663993605e-05, 9.949676788210225e-05, 0.00011348417634772737, 5.789598395396377e-05, 5.636208291119002e-05, 0.00012141526245659619, 0.00012935765334103492, 2.495846196835918e-05, 6.470154347091956e-05, 0.0001218714625828524, 0.0001044306362020955, 3.883853891146619e-05, 7.84091905731201e-05, 0.00010439640342375441, 5.939001056777696e-05, 9.255093128366023e-05, 5.660847225609925e-05, 4.9972528722012964e-05, 8.949477087784792e-05, 8.459018062073713e-05, 5.7738240413584726e-05, 7.92753009390192e-05, 8.313948391090858e-05, 3.104034489963806e-05, 3.4922576519871856e-05, 2.6463805677840565e-05, 6.250103292553367e-05, 5.604349771808582e-05, 1.88850331341025e-05, 5.8078680196711065e-05, 6.984409871092298e-05, 7.95380931768891e-05, 6.807802386435105e-05, 5.9558140436214085e-05, 7.213971585300156e-05, 0.00010742956381038589, 5.608720604574932e-05, 5.297999269479671e-05, 5.636252081641768e-05, 4.2765736927046717e-05, 7.929207579677481e-05, 5.170054352031662e-05, 3.235844291132538e-05, 7.189127482591416e-05, 5.9485339850344885e-05, 2.2872227746178528e-05, 9.034371069921884e-06, 3.370541701959574e-05, 2.0341990707233336e-05, 6.485112257081139e-05, 9.730721318653941e-05, 0.00013873490379153012, 6.815977787487433e-05, 6.730183298348057e-05, 4.0830836888972415e-05, 5.6950738439967104e-06, 3.378526679093192e-05, 5.783801512336395e-05, 0.00011130273912585958, 7.37316408538385e-05, 8.717100093151282e-05, 4.2391260742172246e-05, 9.640844437892159e-05, 0.00010896010978726657, 4.063961127776657e-05, 5.8592322316166396e-05, 9.832190134104383e-05, 7.784131189198688e-05, 7.339203779891448e-05, 8.052290444603476e-05, 5.254474607529348e-05, 1.6934990974464035e-05, 6.473913076511907e-05, 1.2253368037900021e-05, 9.137512258302066e-05, 0.0001121488414027969, 8.571449679469415e-05, 2.6091871960842114e-05, 0.0001303018666404853, 7.20433056337579e-05, 6.249695845606734e-06, 5.489101064908021e-05, 7.039293880441748e-05, 6.844346660738281e-05, 3.243799103428434e-05, 5.122963053040751e-05, 9.277836772132665e-05, 9.663316816260325e-05, 9.047055517785077e-05, 5.313887628073664e-05, 7.291040988571511e-05, 3.123093674094989e-05, 1.6902181789714648e-05, 5.8728408015545155e-05, 3.3124873390271e-05, 2.7698820224219902e-05, 0.00010837994080925189, 0.00014288382367119351, 6.5139745755687e-05, 2.998039199004387e-05, 5.562833455792361e-05, 9.781954934865145e-05, 0.00012007322323158979, 9.328482781678234e-05, 6.240056137756578e-05, 6.58169551672311e-05, 6.12327487763538e-05, 2.817537422284425e-05, 1.7917150359805564e-05, 1.739665383825207e-05, 2.8118451033007985e-06, 2.6522798148353122e-05, 6.631545781670024e-05, 5.165684024618699e-05, 2.1631026538407133e-05, 1.1809912122062645e-06, 3.8807377305429504e-05, 8.913030111518458e-05, 9.70204491874142e-05, 7.412257848450545e-05, 5.8034736074653764e-05, 6.92480484683944e-05, 4.836615311561655e-05, 3.786108395810475e-05, 7.778360935110772e-05, 9.985966569416114e-05, 6.592200902834201e-05, 3.251398386722715e-05, 8.960290062200105e-05, 0.0001342295460552666, 0.0001589347808199238, 0.00012586143570128094, 7.762763233104493e-05, 6.242986028726998e-05, 4.88555914538052e-05, 3.827872144358987e-05, 3.1267453273230836e-05, 1.6626235169223447e-05, 3.828848833350613e-05, 4.694971005164314e-05, 0.000101184054728353, 0.000182784623312052, 0.00016163841824241604, 5.548112411903441e-05, 7.191554604936042e-05, 2.713661483731405e-05, 8.234636339507204e-05, 7.789460847959719e-05, 5.8431089279906395e-05, 0.00010351660014206386, 9.212425351375383e-05, 6.281782578978951e-05, 2.9572266772697958e-05, 0.00011954893594033768, 0.0002466339638049367, 0.00017645789879917187, 8.086077112416246e-05, 0.00011649862570561313, 0.00010676502194584346, 4.379470710757741e-05, 2.992337493656947e-05, 1.707268961008472e-05, 1.093855233850776e-05, 1.728294165919905e-05, 5.3555638739388283e-05, 3.3636160153926004e-05, 2.7048489615121222e-05, 5.552535854710012e-05, 3.5083616718634565e-05, 0.000113775469576003, 7.942127126999557e-05, 3.543442824298634e-05, 5.045362377409201e-05, 0.00016534046136717142, 0.00018311315284389346, 6.429406871878587e-05, 1.732298024604163e-05, 9.352489697415701e-05, 0.00019664270839550476, 0.00018165653164511653, 6.744277337521831e-05, 2.4156228945603937e-05, 7.857838172448876e-05, 9.338578546972164e-05, 7.251833357484212e-05, 4.103191180296767e-05, 4.4601976834397864e-05, 5.581693629735729e-05, 3.509515954301607e-05, 2.2575159437128305e-05, 4.3728589582796625e-05]}
  out "Raw Voltage (FFT)":cluster{"f0":dbl, "df":dbl, "magnitude":dbl[]}(graph)
  out "Raw I & V":waveform(dbl)[](graph)
  in  "Tab Control":enum32{"Inputs", "Status", "Output"}(tab)
  in  "Error In (No Error)":errorcluster
  out "Signal Average #":i32
  out "Mean Current":dbl format="%0.2f"
  out "Mean Voltage":dbl format="%0.2f"
  out "Sample Multiplier":i32
  out "Characters Read":string
  out "Pre-Check Active":bool
  out "Pre-Check Pot Instr Error":errorcluster
  out "dt (DAQ)":dbl
  out "Final Sampling Rate":dbl
  out "Data Size (low freq)":dbl
  out "Data Size":dbl
  out "Pre-Check (Real-Time)":dbl(graph)
  out "wfm info":T1(array[cluster]) caption="NISCOPE wfm info" {"reserved2" format="%.2f"; "reserved1" format="%.2f"; "offset" format="%^.3e"; "gain" format="%^.3e"; "xIncrement" format="%^.3e"; "relativeInitialX" format="%^.3e"; "absoluteInitialX" format="%^.3e"}
  out "Output Data Array":dbl[][](array[numeric])
  # "Raw DAQ Output"
  # "Post Low-Freq Filtering"
  # "Post Signal Averaging"
  # "Raw DAQ Output (FFT)"
  # "Post Signal Averaging"
  # "Sweep Progress"
  # "Sampling Info"
  # "Signal Averaging"
  # "Bias Reject"
  # "Pre-Check"
  # "DAQ Settings"
  # "Write to File"
  # "Sampling Info"
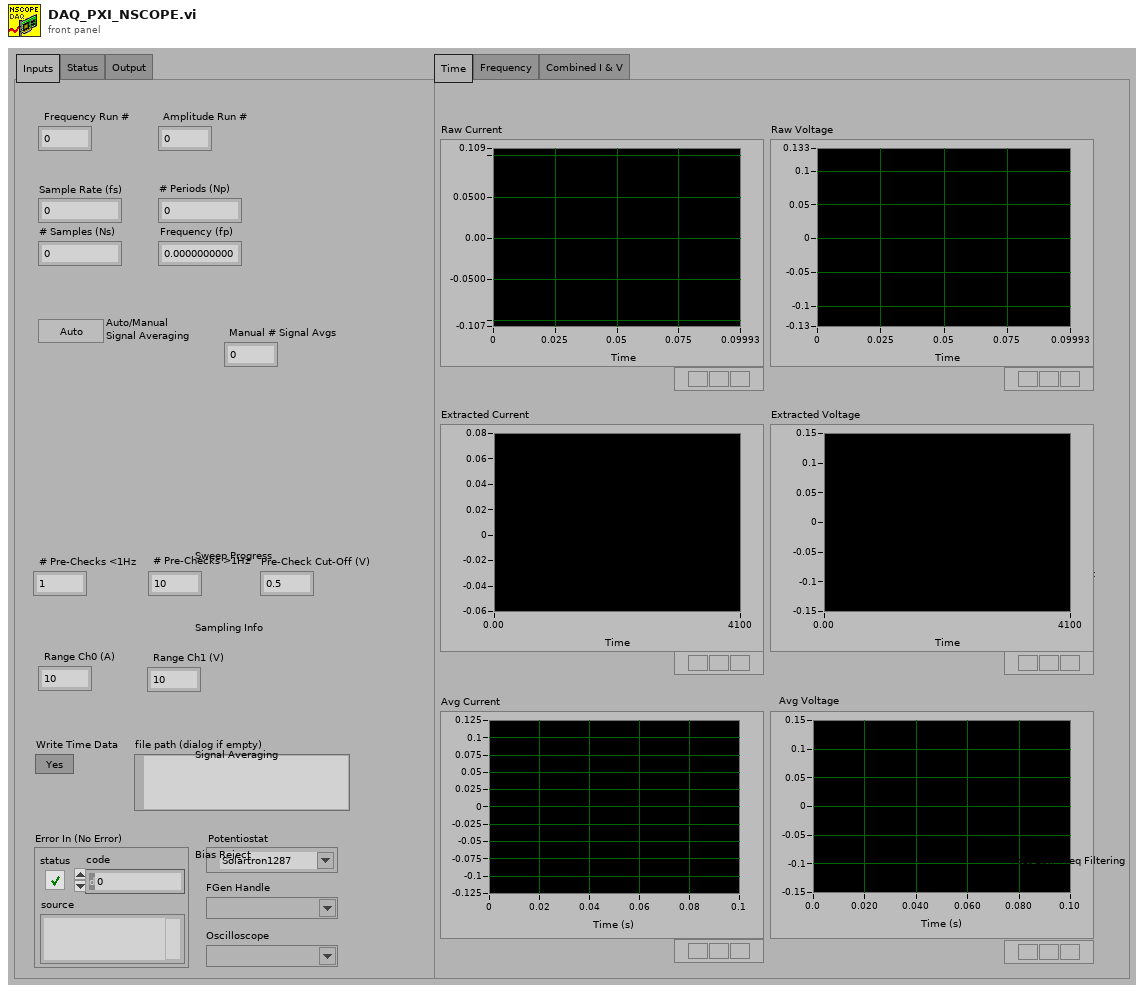
[diagram p1: front panel]
types:
  T1 = cluster{"actualSamples":i32, "absoluteInitialX":dbl, "relativeInitialX":dbl, "xIncrement":dbl, "offset":dbl, "gain":dbl, "reserved1":dbl, "reserved2":dbl}[]
  T2 = typedef "niScope trigger source digital.ctl" = string
  T3 = typedef "niScope timestamp type.ctl" = i32
  T4 = typedef "niScope trigger slope.ctl" = i32
  T5 = enum16{"None ", "Hanning", "Hamming", "Blackman-Harris", "Exact Blackman", "Blackman", "Flat Top", "4 Term B-Harris ", "7 Term B-Harris", "Low Sidelobe"}
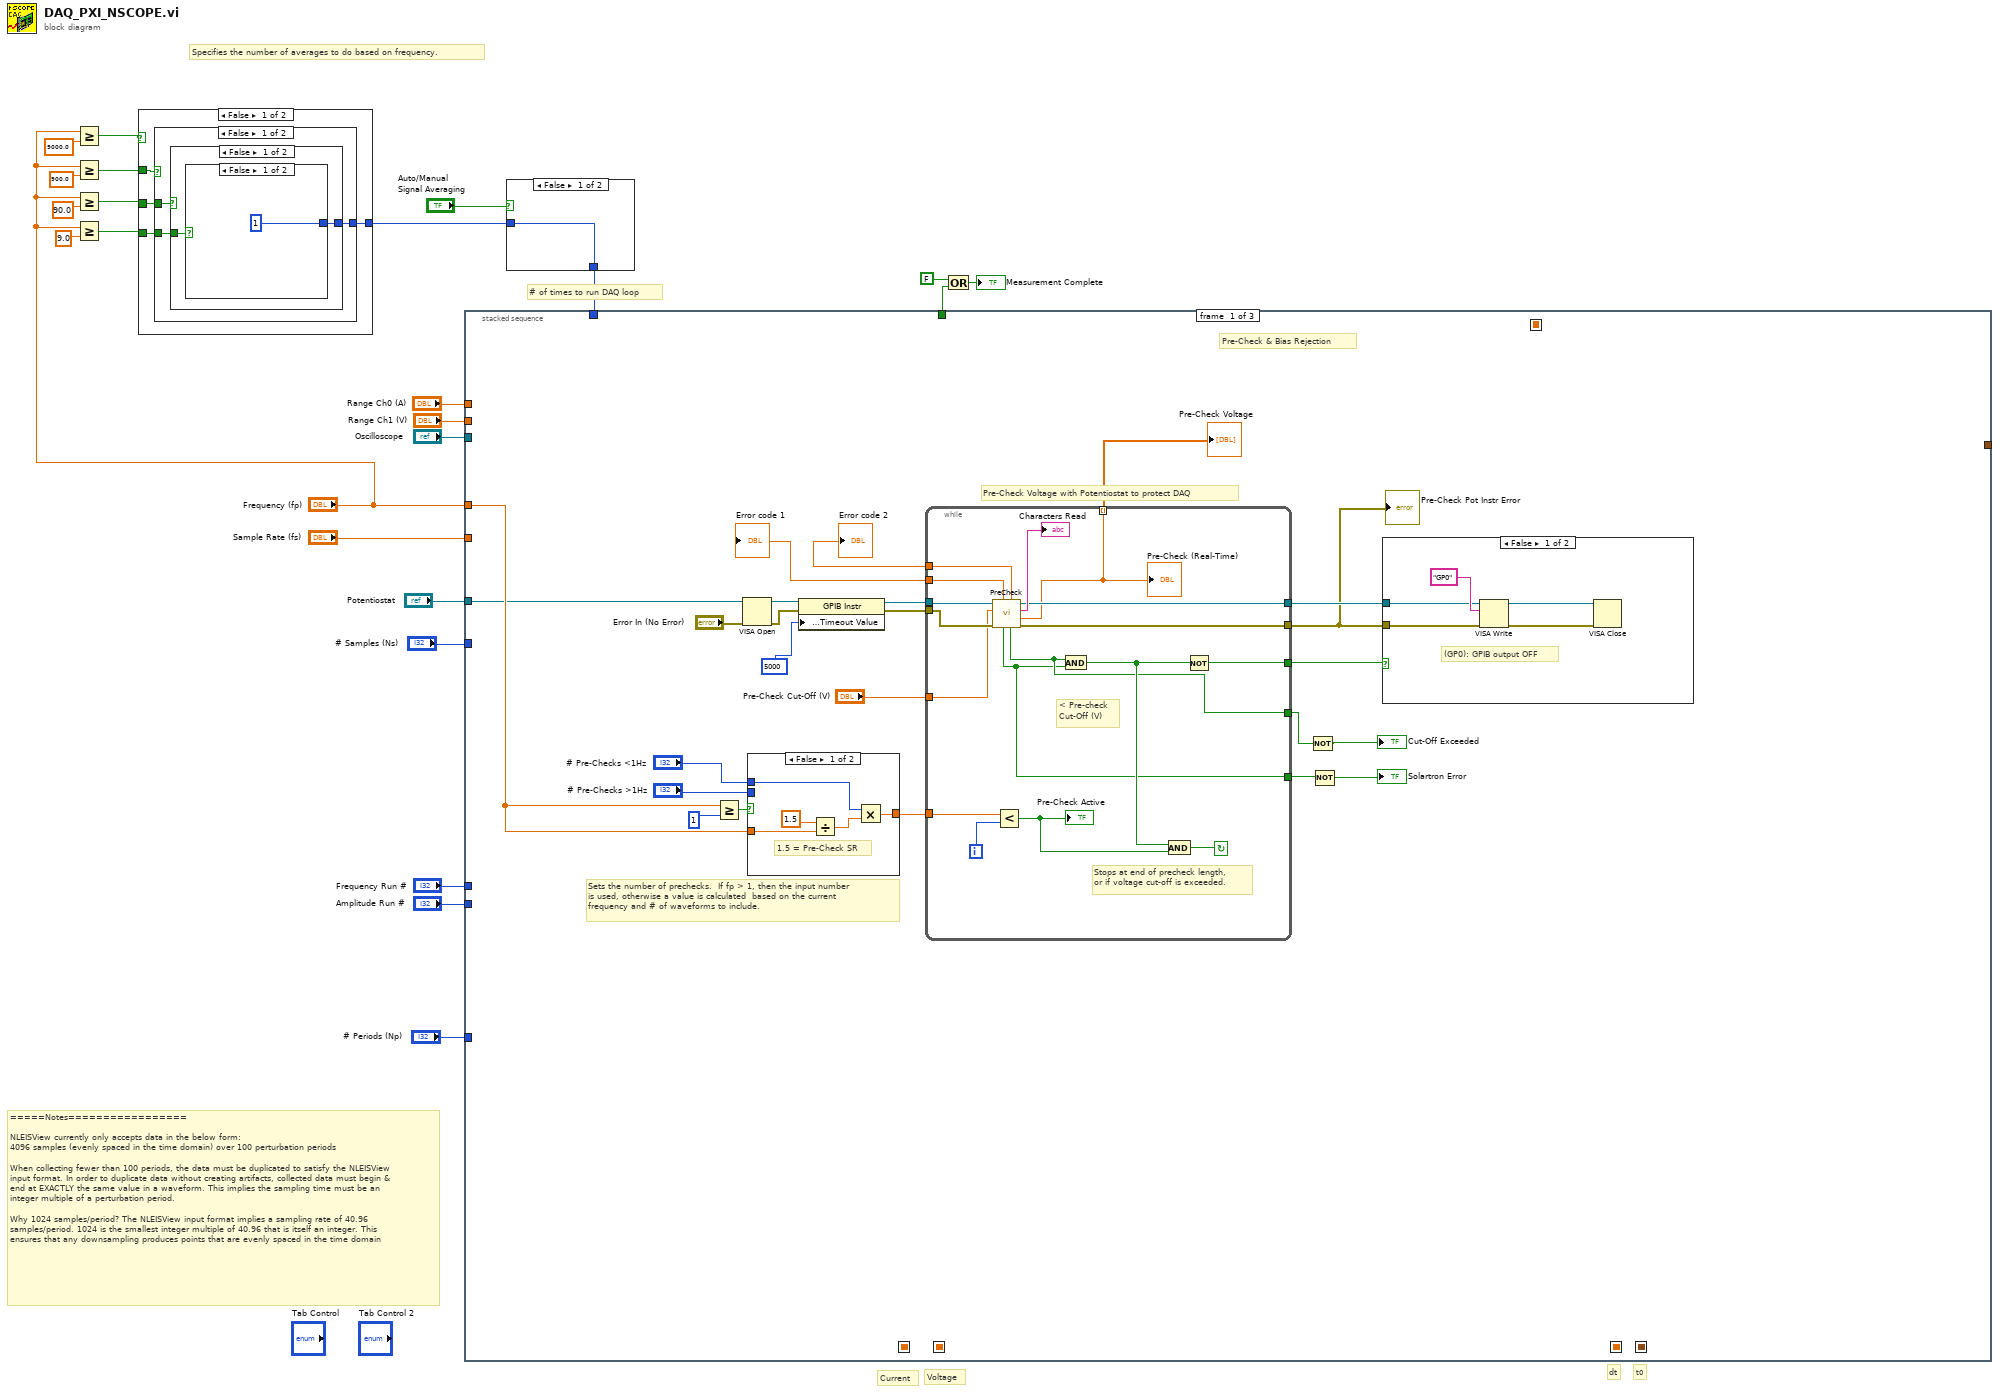
[diagram p0: block diagram]
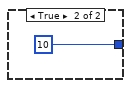
[diagram p2: hidden frame]
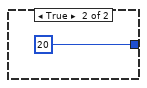
[diagram p3: hidden frame]
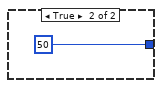
[diagram p4: hidden frame]
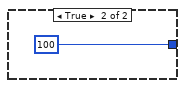
[diagram p5: hidden frame]
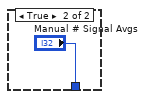
[diagram p6: hidden frame]
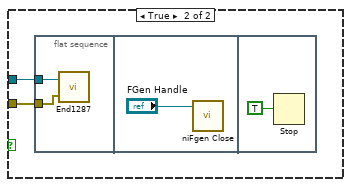
[diagram p7: hidden frame]
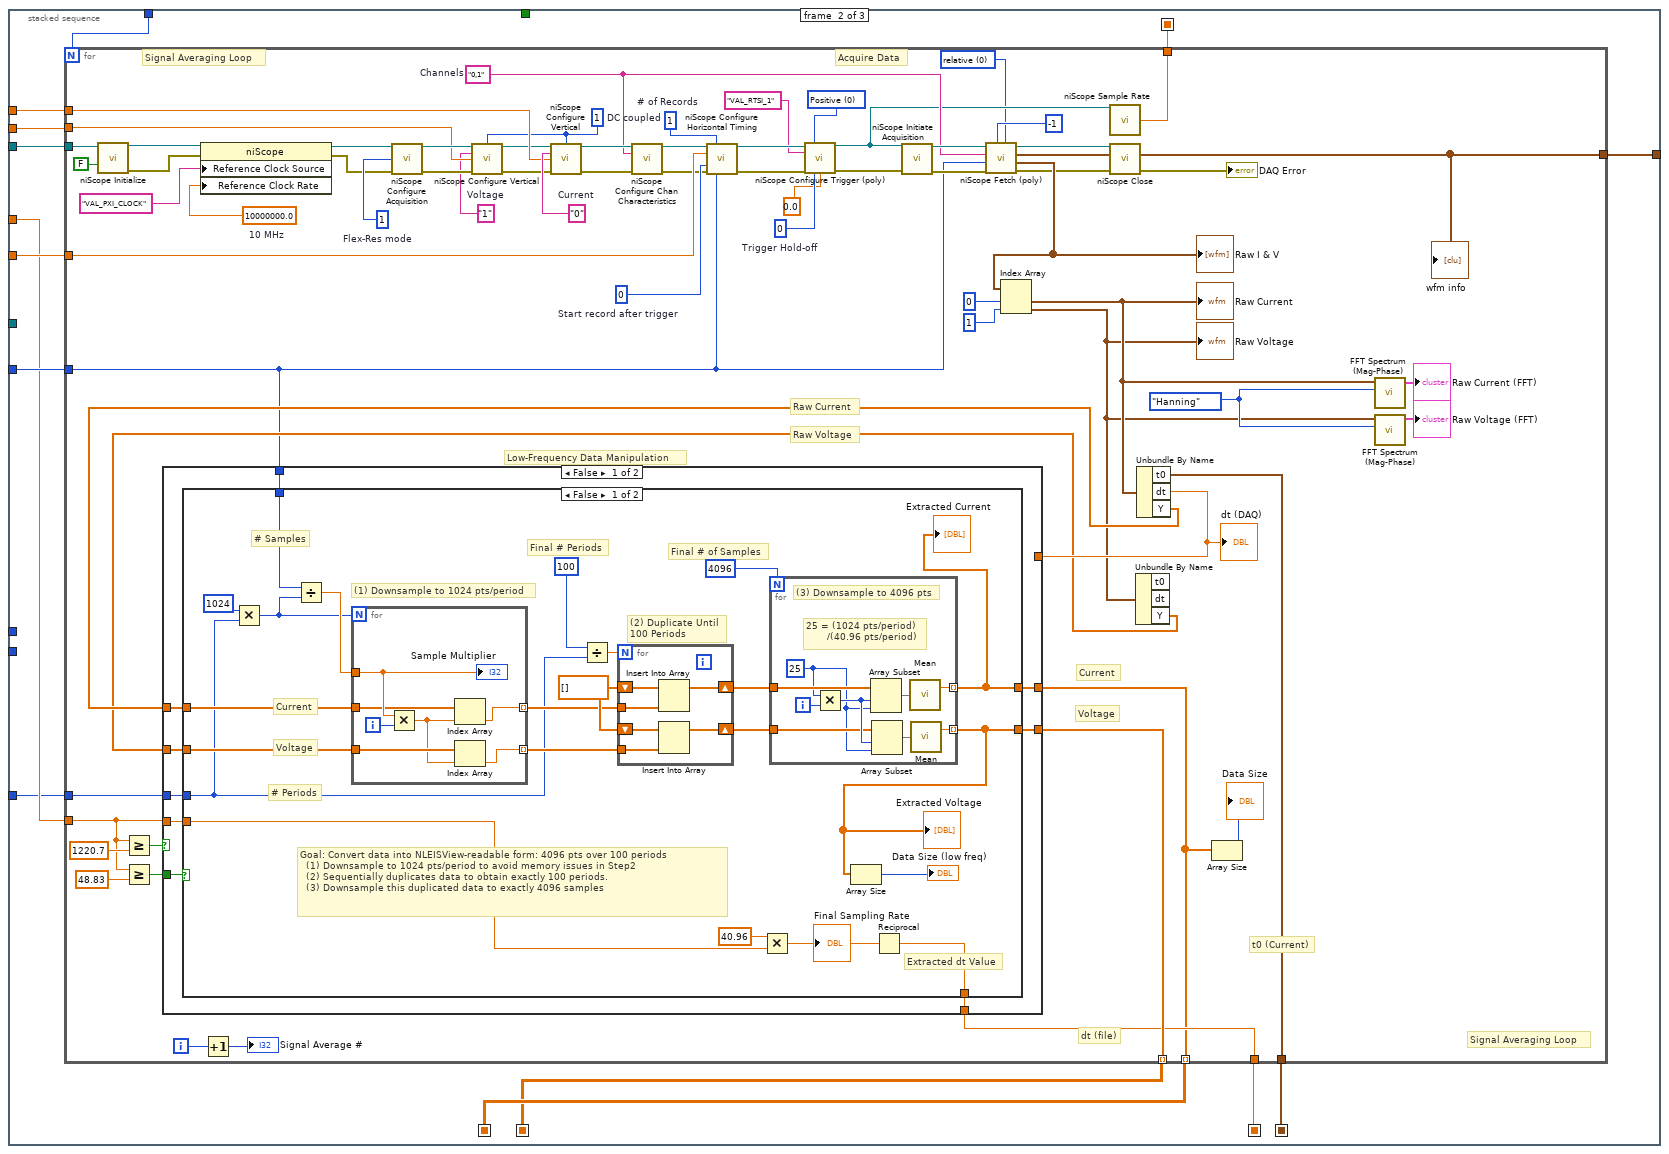
[diagram p9: hidden frame]
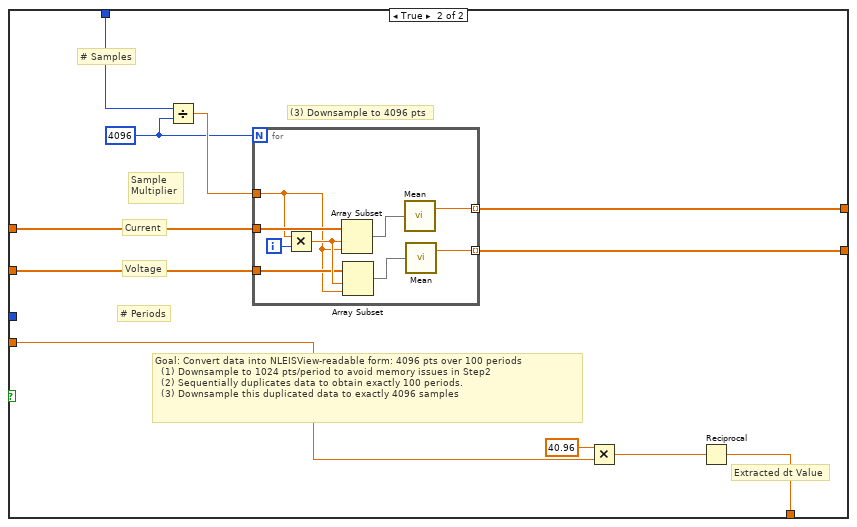
[diagram p10: hidden frame]
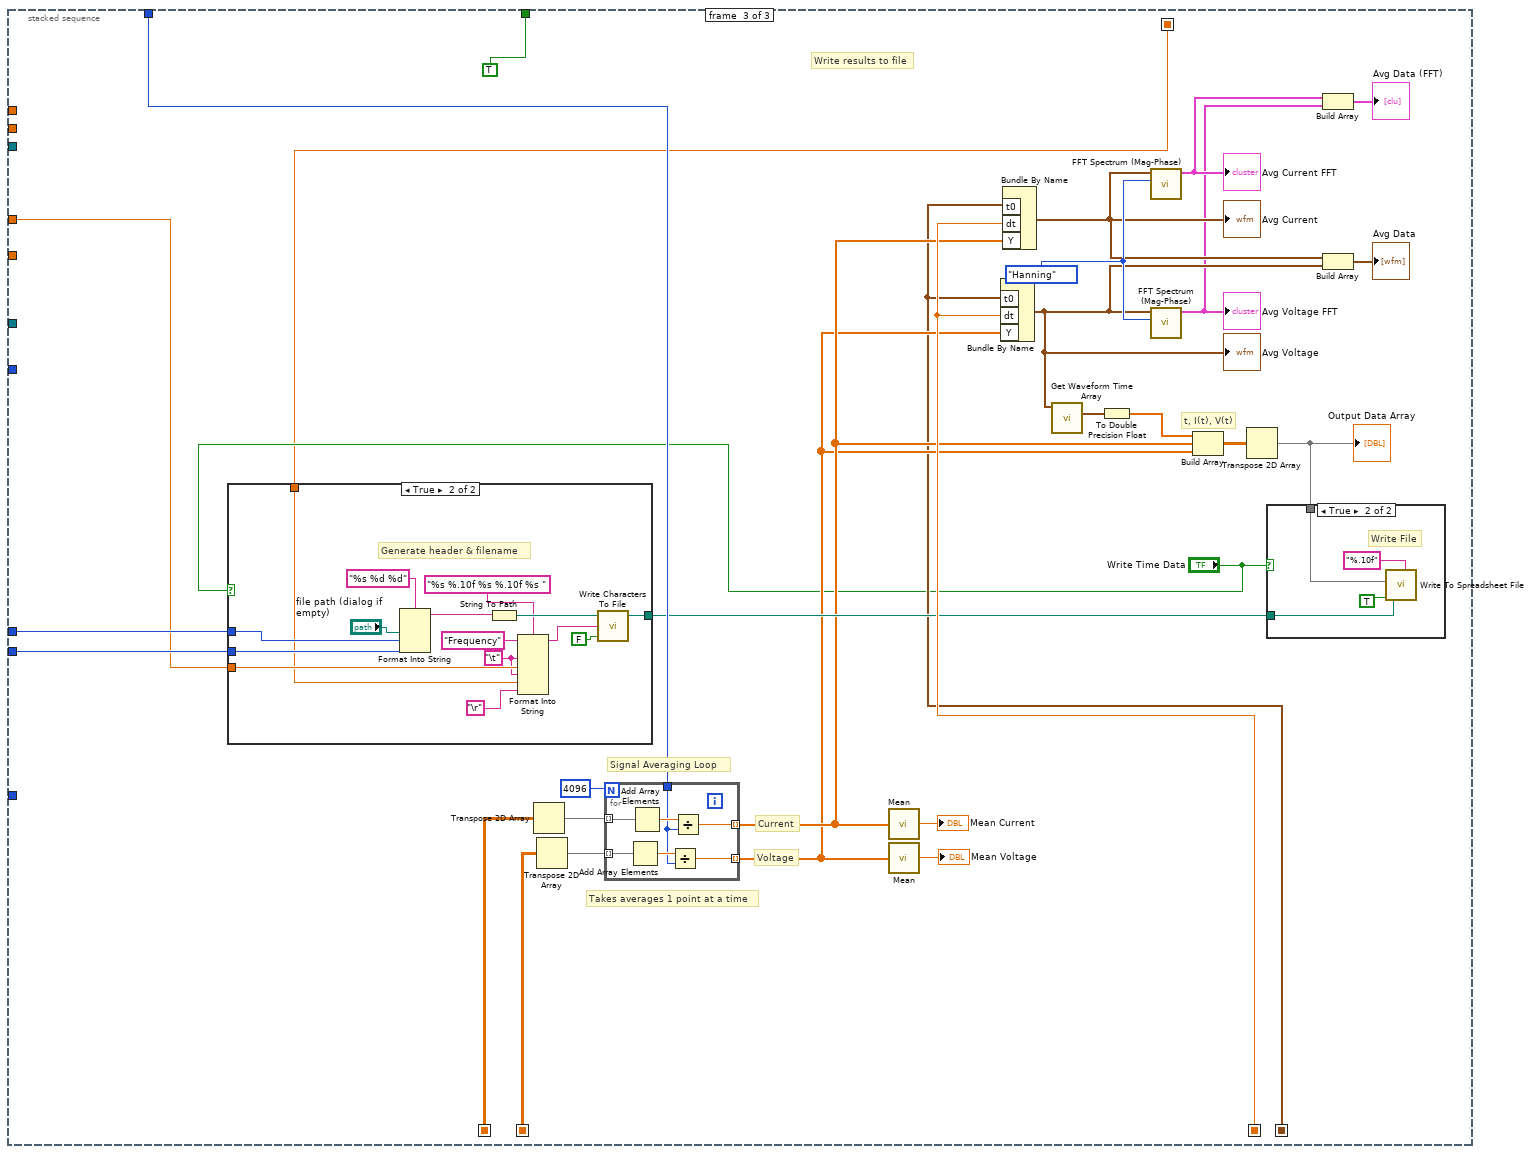
[diagram p12: hidden frame]
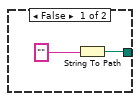
[diagram p13: hidden frame]
diagram:
  # "# of times to run DAQ loop"
  # "=====Notes=================\n\nNLEISView currently only accepts data in the below form:\n4096 samples (evenly spaced in the time domain) over 100 perturbation periods\n\nWhen collecting fewer than 100 periods, the data must be duplicated to satisfy the NLEISView input format. In order to duplicate data without creating artifacts, collected data must begin & end at EXACTLY the same value in a waveform. This implies the sampling time must be an integer multiple of a perturbation period.\n\nWhy 1024 samples/period? The NLEISView input format implies a sampling rate of 40.96 samples/period. 1024 is the smallest integer multiple of 40.96 that is itself an integer. This ensures that any downsampling produces points that are evenly spaced in the time domain"
  # "Specifies the number of averages to do based on frequency."
  # "t0"
  # "dt"
  # "Voltage"
  # "Current"
  n1 = Greater Or Equal?(x="Frequency (fp)", y=9000.0) -> (x >= y?=w7:bool)
  n2 = Greater Or Equal?(x="Frequency (fp)", y=900.0) -> (x >= y?=w6:bool)
  n3 = Greater Or Equal?(x="Frequency (fp)", y=90.0) -> (x >= y?=w5:bool)
  n4 = Greater Or Equal?(x="Frequency (fp)", y=9.0) -> (x >= y?=w4:bool)
  n5 = case shown="False" w7 {
    tunnel: w5 -> [w27 _]
    tunnel: w4 -> [w26 _]
    tunnel: [w28 100 ("x")] -> w3
    tunnel: w6 -> [w25 _]
    frame False {
      n6 = case shown="False" w25 {
        tunnel: [w30 50 ("x")] -> w28
        tunnel: w27 -> [w31 _]
        tunnel: w26 -> [w29 _]
        frame False {
          n7 = case shown="False" w31 {
            tunnel: [w32 20 ("x")] -> w30
            tunnel: w29 -> [w33 _]
            frame False {
              n8 = case shown="False" w33 {
                tunnel: [1 ("x") 10 ("x")] -> w32
                frame False {
                }
                frame True {
                }
              }
            }
            frame True {
            }
          }
        }
        frame True {
        }
      }
    }
    frame True {
    }
  }
  n9 = case shown="False" "Auto/Manual \nSignal Averaging" {
    tunnel: w3 -> [w39 _]
    tunnel: [w39 "Manual # Signal Avgs"] -> w13
    frame False {
    }
    frame True {
    }
  }
  n10 = stacked-sequence {
    seq-local: [_ w112 _] -> [_ _ w282]
    seq-local: [_ w111 _] -> [_ _ w285]
    seq-local: [_ w107 _] -> [_ _ w279]
    seq-local: [_ w106 _] -> [_ _ w259]
    seq-local: [_ w99 _] -> [_ _ w257]
    tunnel: "Range Ch0 (A)" -> [_ w110 _]
    tunnel: w13 -> [_ w109 w280]
    tunnel: "Amplitude Run #" -> [_ _ w281]
    tunnel: "Range Ch1 (V)" -> [_ w108 _]
    tunnel: "Sample Rate (fs)" -> [_ w105 _]
    tunnel: "# Samples (Ns)" -> [_ w104 _]
    tunnel: "Frequency (fp)" -> [w64 w103 w270]
    tunnel: "# Periods (Np)" -> [_ w102 _]
    tunnel: [_ _ TRUE] -> w22
    tunnel: "Frequency Run #" -> [_ _ w275]
    tunnel: "Potentiostat" -> [w63 _ _]
    tunnel: "Oscilloscope" -> [_ w101 _]
    tunnel: [_ w100 _] -> _
    frame #0 {
      # "Sets the number of prechecks.  If fp > 1, then the input number \nis used, otherwise a value is calculated  based on the current \nfrequency and # of waveforms to include."
      # "Pre-Check Voltage with Potentiostat to protect DAQ"
      # "Pre-Check & Bias Rejection"
      n11 = Greater Or Equal?(x=w64, y=1) -> (x >= y?=w62:bool)
      n12 = VISA Open(error in (no error)="Error In (No Error)", VISA resource name=w63) -> (VISA resource name=w56:refnum<visa-resource-name>, error out=w55:errorcluster)  [unwired: 3 in]
      n13 = case shown="False" w62 {
        tunnel: w64 -> [w93 _]
        tunnel: [w95 w98] -> w52
        tunnel: "# Pre-Checks >1Hz" -> [_ w98]
        tunnel: "# Pre-Checks <1Hz" -> [w94 _]
        frame False {
          # "1.5 = Pre-Check SR"
          n14 = Divide(x=1.5, y=w93) -> (x/y=w96:dbl)
          n15 = Multiply(x=w94, y=w96) -> (x*y=w95:dbl)
        }
        frame True {
        }
      }
      n16 = property class="GPIB Instr"(reference=w56, error in=w55, "General Settings:Timeout Value"=u32 5000) -> (reference out=w54:refnum<visa-resource-name>, error out=w53:errorcluster)
      n17 = while {
        tunnel: w52 -> [w91]
        tunnel: [w89] -> w49
        tunnel: w54 -> [w87]
        tunnel: w53 -> [w86]
        tunnel: "Pre-Check Cut-Off (V)" -> [w85]
        tunnel: [w83] -> w50
        tunnel: [w82] -> w48
        tunnel: [w81] -> w47 mode=indexing
        tunnel: [w79] -> w46
        tunnel: [w78] -> w45
        tunnel: [w77] -> w44
        tunnel: [w76] -> w42
        i -> [w92]
        stop <- w90 continue-if-true
        # "Stops at end of precheck length,\nor if voltage cut-off is exceeded."
        # "< Pre-check\nCut-Off (V)"
        n18 = call "PreCheck.vi"("Error In (No Error)"=w86, "Pre-Check Cut-Off (V)"=w85, "Potentiostat"=w87) -> ("Error Out"=w82:errorcluster, "Pre-Check Voltage"=w81:dbl, "Characters Read"=→"Characters Read":string, "Potentiostat"=w83:refnum<visa-resource-name>, "<Cut-Off?"=w77:bool, "Error code 2"=w78:dbl, "No potentiostat Error?"=w76:bool, "Error code 1"=w79:dbl)  [unwired: 1 in]
        "Pre-Check (Real-Time)" <- w81
        n19 = Less?(x=w92, y=w91) -> (x < y?=w88:bool)
        "Pre-Check Active" <- w88
        n20 = And(x=w77, y=w76) -> (x .and. y?=w80:bool)
        n21 = And(x=w80, y=w88) -> (x .and. y?=w90:bool)
        n22 = Not(x=w80) -> (.not. x?=w89:bool)
      }
      "Pre-Check Pot Instr Error" <- w48
      "Pre-Check Voltage" <- w47
      "Error code 1" <- w46
      "Error code 2" <- w45
      n23 = Not(x=w44) -> (.not. x?=→"Cut-Off Exceeded":bool)
      n24 = Not(x=w42) -> (.not. x?=→"Solartron Error":bool)
      n25 = case shown="False" w49 {
        tunnel: w50 -> [w68 w70]
        tunnel: w48 -> [w67 w71]
        frame False {
          # "(GP0): GPIB output OFF"
          n26 = VISA Write(VISA resource name=w68, write buffer="GP0" ("Characters to Write"), error in (no error)=w67) -> (VISA resource name out=w66:refnum<visa-resource-name>, error out=w65:errorcluster)  [unwired: 1 out]
          n27 = VISA Close(VISA resource name=w66, error in (no error)=w65) -> ()  [unwired: 1 out]
        }
        frame True {
          n28 = flat-sequence {
            tunnel: w70 -> [w72]
            tunnel: w71 -> [w73]
            frame #0 {
              n29 = call "End1287.vi"("Error In (No Error)"=w73, "VISA Name In"=w72) -> ()  [unwired: 2 out]
            }
            frame #1 {
              n30 = call <instrlib>:"niFgen Close.vi"("Instrument Handle"="FGen Handle") -> ()  [unwired: 10 in, 1 out]
            }
            frame #2 {
              n31 = Stop(stop? (T)=TRUE) -> ()
            }
          }
        }
      }
    }
    frame #1 {
      n32 = for {
        N: w109 -> [_]
        tunnel: [w169] -> w112 mode=indexing
        tunnel: [w175] -> w111 mode=indexing
        tunnel: w110 -> [w134]
        tunnel: w104 -> [w149]
        tunnel: w108 -> [w129]
        tunnel: [w174] -> w107
        tunnel: [w165] -> w106
        tunnel: w105 -> [w155]
        tunnel: w103 -> [w138]
        tunnel: w102 -> [w171]
        tunnel: w101 -> [w141]
        tunnel: [w136] -> w100
        tunnel: [w114] -> w99
        i -> [w173]
        w113 = T3 0 items=["relative", "absolute"] ("timestamp Type")
        w118 = T4 0 items=["Positive", "Negative"] ("trigger slope")
        w128 = "1"  # Voltage
        w135 = "0"  # Current
        w144 = 10000000.0  # 10 MHz
        w154 = 0  # Trigger Hold-off
        w158 = 0  # Start record after trigger
        w159 = 1  # # of Records
        w127 = 1  # DC coupled
        w119 = "0,1"  # Channels
        w160 = 1  # Flex-Res mode
        w180 = T5."Hanning" ("window")
        # "Acquire Data"
        # "Signal Averaging Loop"
        # "Signal Averaging Loop"
        # "t0 (Current)"
        # "dt (file)"
        # "Raw Voltage"
        # "Raw Current"
        # "Voltage"
        # "Current"
        # "Low-Frequency Data Manipulation"
        n33 = call <instrlib>:"niScope Initialize.vi"("resource name"=w141, "reset device"=FALSE) -> ("instrument handle"=w143:refnum<k15>, "error out"=w142:errorcluster)  [unwired: 12 in]
        n34 = Greater Or Equal?(x=w138, y=1220.7) -> (x >= y?=w167:bool)
        n35 = Greater Or Equal?(x=w138, y=48.83) -> (x >= y?=w137:bool)
        n36 = property class="niScope"(reference=w143, error in=w142, "Reference Clock Source"="VAL_PXI_CLOCK" ("Source"), "Reference Clock Rate"=w144) -> (reference out=w125:refnum<k15>, error out=w124:errorcluster)
        n37 = Increment(x=w173) -> (x+1=→"Signal Average #":i32)
        n38 = call <instrlib>:"niScope Configure Acquisition.vi"("instrument handle"=w125, "acquisition Type"=w160, "error in"=w124) -> ("instrument handle out"=w133:refnum<k15>, "error out"=w131:errorcluster)  [unwired: 11 in]
        n39 = call <instrlib>:"niScope Configure Vertical.vi"("instrument handle"=w133, "vertical coupling"=w127, "channels"=w128, "vertical range"=w129, "error in"=w131) -> ("instrument handle out"=w132:refnum<k15>, "error out"=w130:errorcluster)  [unwired: 9 in]
        n40 = call <instrlib>:"niScope Configure Vertical.vi"("instrument handle"=w132, "vertical coupling"=w127, "channels"=w135, "vertical range"=w134, "error in"=w130) -> ("instrument handle out"=w123:refnum<k15>, "error out"=w121:errorcluster)  [unwired: 9 in]
        n41 = call <instrlib>:"niScope Configure Chan Characteristics.vi"("instrument handle"=w123, "channels"=w119, "error in"=w121) -> ("instrument handle out"=w122:refnum<k15>, "error out"=w120:errorcluster)  [unwired: 11 in]
        n42 = call <instrlib>:"niScope Configure Horizontal Timing.vi"("instrument handle"=w122, "number of records"=w159, "min sample rate"=w155, "reference position"=w158, "error in"=w120, "min record length"=w149) -> ("instrument handle out"=w157:refnum<k15>, "error out"=w156:errorcluster)  [unwired: 8 in]
        n43 = call-poly <instrlib>:"niScope Configure Trigger (poly).vi"("instrument handle"=w157, "trigger slope"=w118, "trigger source"=T2 "VAL_RTSI_1", "error in"=w156, "trigger holdoff"=w154, "trigger delay"=0.0) -> ("instrument handle out"=w115:refnum<k15>, "error out"=w153:errorcluster)  [unwired: 8 in]
        n44 = call <instrlib>:"niScope Initiate Acquisition.vi"("instrument handle"=w115, "error in"=w153) -> ("instrument handle out"=w152:refnum<k15>, "error out"=w151:errorcluster)  [unwired: 12 in]
        n45 = call-poly <instrlib>:"niScope Fetch (poly).vi"("timestamp Type"=w113, "timeout"=-1, "error in"=w151, "numSamples"=w149, "channels"=w119, "instrument handle"=w152) -> ("error out"=w147:errorcluster, "wfm"=w148:waveform(dbl)[], "wfm info"=w136:T1, "instrument handle out"=w146:refnum<k15>)  [unwired: 2 in]
        "Raw I & V" <- w148
        "wfm info" <- w136
        n46 = Index Array(array=w148, index #1=0 ("index"), index #2=1 ("index")) -> (element #1=w162:waveform(dbl), element #2=w161:waveform(dbl))
        "Raw Current" <- w162
        "Raw Voltage" <- w161
        n47 = call <instrlib>:"niScope Sample Rate.vi"("instrument handle"=w115) -> ("actual sample rate"=w114:dbl)  [unwired: 12 in, 2 out]
        n48 = call <instrlib>:"niScope Close.vi"("instrument handle"=w146, "error in"=w147) -> ("error out"=→"DAQ Error":errorcluster)  [unwired: 13 in]
        n49 = Unbundle By Name(w161) -> ("Y"=w163:dbl[])  [unwired: 2 out]
        n50 = Unbundle By Name(w162) -> ("t0"=w165:timestamp, "dt"=w166:dbl, "Y"=w164:dbl[])
        "dt (DAQ)" <- w166
        n51 = case shown="False" w167 {
          tunnel: [w188 w256] -> w169
          tunnel: w164 -> [w187 w256]
          tunnel: w163 -> [w186 w255]
          tunnel: [w184 w255] -> w175
          tunnel: w138 -> [w185 _]
          tunnel: [w189 w254] -> w174
          tunnel: w166 -> [_ w254]
          tunnel: w171 -> [w182 _]
          tunnel: w149 -> [w183 _]
          tunnel: w137 -> [w181 _]
          frame False {
            n52 = case shown="False" w181 {
              tunnel: [w211 w237] -> w189
              tunnel: [w210 w235] -> w188
              tunnel: w187 -> [w205 w240]
              tunnel: w186 -> [w204 w239]
              tunnel: w185 -> [w201 w238]
              tunnel: [w199 w234] -> w184
              tunnel: w183 -> [w193 w241]
              tunnel: w182 -> [w192 _]
              frame False {
                w208 = dbl[] []
                # "# Samples"
                # "Voltage"
                # "Current"
                # "Final # Periods"
                # "# Periods"
                # "Final # of Samples"
                # "(1) Downsample to 1024 pts/period"
                # "(2) Duplicate Until \n100 Periods"
                # "Goal: Convert data into NLEISView-readable form: 4096 pts over 100 periods\n  (1) Downsample to 1024 pts/period to avoid memory issues in Step2\n  (2) Sequentially duplicates data to obtain exactly 100 periods.\n  (3) Downsample this duplicated data to exactly 4096 samples"
                # "Extracted dt Value"
                n53 = Multiply(x=1024 ("element"), y=w192) -> (x*y=w190:i32)
                n54 = Divide(x=w193, y=w190) -> (x/y=w191:dbl)
                n55 = for {
                  N: w190 -> [_]
                  tunnel: w191 -> [w217]
                  tunnel: w205 -> [w216]
                  tunnel: [w215] -> w203 mode=indexing
                  tunnel: w204 -> [w214]
                  tunnel: [w212] -> w202 mode=indexing
                  i -> [w218]
                  n56 = Multiply(x=w217, y=w218) -> (x*y=w213:dbl)
                  n57 = Index Array(array=w216, index=w213) -> (element=w215:dbl)
                  n58 = Index Array(array=w214, index=w213) -> (element=w212:dbl)
                  "Sample Multiplier" <- w217
                }
                n59 = Divide(x=100 ("y"), y=w192) -> (x/y=w209:dbl)
                n60 = for {
                  N: w209 -> [_]
                  shift-right: [w222] -> w207
                  shift-left: w208 -> [w224]
                  shift-right: [w219] -> w206
                  shift-left: w208 -> [w221]
                  tunnel: w203 -> [w223]
                  tunnel: w202 -> [w220]
                  n61 = Insert Into Array(array=w224, new element=w223) -> (w222:dbl[])  [unwired: 1 in]
                  n62 = Insert Into Array(array=w221, new element=w220) -> (w219:dbl[])  [unwired: 1 in]
                }
                n63 = Multiply(x=40.96 ("y"), y=w201) -> (x*y=w196:dbl)
                "Final Sampling Rate" <- w196
                n64 = for {
                  N: 4096 ("element") -> [_]
                  tunnel: w207 -> [w233]
                  tunnel: [w230] -> w210 mode=indexing
                  tunnel: w206 -> [w231]
                  tunnel: [w229] -> w199 mode=indexing
                  i -> [w228]
                  w225 = 25 ("element")
                  # "(3) Downsample to 4096 pts"
                  # "25 = (1024 pts/period)\n       /(40.96 pts/period)"
                  n65 = Multiply(x=w225, y=w228) -> (x*y=w232:i32)
                  n66 = Array Subset(array=w233, index=w232, length=w225) -> (w227:dbl[])
                  n67 = Array Subset(array=w231, index=w232, length=w225) -> (w226:dbl[])
                  n68 = call-poly <vilib>:"Mean.vi"("X"=w227) -> ("mean"=w230:dbl)  [unwired: 1 out]
                  n69 = call-poly <vilib>:"Mean.vi"("X"=w226) -> ("mean"=w229:dbl)  [unwired: 1 out]
                }
                "Extracted Current" <- w210
                "Extracted Voltage" <- w199
                n70 = Array Size(array=w199) -> (size(s)=→"Data Size (low freq)":i32)
                n71 = Reciprocal(x=w196) -> (1/x=w211:dbl)
              }
              frame True {
                w236 = 4096
                # "# Samples"
                # "Sample\nMultiplier"
                # "Voltage"
                # "Current"
                # "# Periods"
                # "(3) Downsample to 4096 pts"
                # "Goal: Convert data into NLEISView-readable form: 4096 pts over 100 periods\n  (1) Downsample to 1024 pts/period to avoid memory issues in Step2\n  (2) Sequentially duplicates data to obtain exactly 100 periods.\n  (3) Downsample this duplicated data to exactly 4096 samples"
                # "Extracted dt Value"
                n72 = Divide(x=w241, y=w236) -> (x/y=w244:dbl)
                n73 = for {
                  N: w236 -> [_]
                  tunnel: w244 -> [w245]
                  tunnel: w240 -> [w253]
                  tunnel: [w250] -> w235 mode=indexing
                  tunnel: w239 -> [w251]
                  tunnel: [w249] -> w234 mode=indexing
                  i -> [w248]
                  n74 = Multiply(x=w245, y=w248) -> (x*y=w252:dbl)
                  n75 = Array Subset(array=w253, index=w252, length=w245) -> (w247:dbl[])
                  n76 = Array Subset(array=w251, index=w252, length=w245) -> (w246:dbl[])
                  n77 = call-poly <vilib>:"Mean.vi"("X"=w247) -> ("mean"=w250:dbl)  [unwired: 1 out]
                  n78 = call-poly <vilib>:"Mean.vi"("X"=w246) -> ("mean"=w249:dbl)  [unwired: 1 out]
                }
                n79 = Multiply(x=40.96 ("y"), y=w238) -> (x*y=w243:dbl)
                n80 = Reciprocal(x=w243) -> (1/x=w237:dbl)
              }
            }
          }
          frame True {
          }
        }
        n81 = Array Size(array=w169) -> (size(s)=→"Data Size":i32)
        n82 = call-poly <vilib>:"FFT Spectrum (Mag-Phase).vi"("window"=w180, "time signal"=w162) -> ("magnitude"=→"Raw Current (FFT)":cluster{"f0":dbl, "df":dbl, "magnitude":dbl[]})  [unwired: 5 in, 4 out]
        n83 = call-poly <vilib>:"FFT Spectrum (Mag-Phase).vi"("window"=w180, "time signal"=w161) -> ("magnitude"=→"Raw Voltage (FFT)":cluster{"f0":dbl, "df":dbl, "magnitude":dbl[]})  [unwired: 5 in, 4 out]
      }
    }
    frame #2 {
      w286 = T5."Hanning" ("window")
      # "Write results to file"
      # "t, I(t), V(t)"
      # "Takes averages 1 point at a time"
      # "Voltage"
      # "Current"
      # "Signal Averaging Loop"
      n84 = case shown="True" "Write Time Data" {
        tunnel: w281 -> [_ w302]
        tunnel: w275 -> [_ w300]
        tunnel: [w288 w295] -> w271
        tunnel: w270 -> [_ w292]
        tunnel: w257 -> [_ w289]
        frame False {
          n85 = String To Path(string="") -> (path=w288:path)
        }
        frame True {
          w291 = "\t"
          # "Generate header & filename"
          n86 = Format Into String(format string="%s %d %d", "file path (dialog if empty)", w300, w302) -> (resulting string=w297:string)  [unwired: 2 in, 1 out]
          n87 = String To Path(string=w297) -> (path=w296:path)
          n88 = Format Into String(format string="%s %.10f %s %.10f %s " ("format (%.3f)"), initial string="Frequency", w291, w292, w291, w289, "\r") -> (resulting string=w298:string)  [unwired: 1 in, 1 out]
          n89 = call <vilib>:"Write Characters To File.vi"("append to file? (new file:F)"=FALSE, "character string"=w298, "file path (dialog if empty)"=w296) -> ("new file path (Not A Path if cancelled)"=w295:path)  [unwired: 2 in]
        }
      }
      n90 = Transpose 2D Array(2D array=w282) -> (transposed array=w283:dbl[][])
      n91 = Transpose 2D Array(2D array=w285) -> (transposed array=w284:dbl[][])
      n92 = for {
        N: 4096 ("element") -> [_]
        tunnel: w284 -> [w314] mode=indexing
        tunnel: w280 -> [w311]
        tunnel: [w310] -> w267 mode=indexing
        tunnel: [w309] -> w268 mode=indexing
        tunnel: w283 -> [w308] mode=indexing
        n93 = Add Array Elements(numeric array=w314) -> (sum=w312:dbl)
        n94 = Add Array Elements(numeric array=w308) -> (sum=w313:dbl)
        n95 = Divide(x=w312, y=w311) -> (x/y=w310:dbl)
        n96 = Divide(x=w313, y=w311) -> (x/y=w309:dbl)
      }
      n97 = call-poly <vilib>:"Mean.vi"("X"=w268) -> ("mean"=→"Mean Current":dbl)  [unwired: 1 out]
      n98 = call-poly <vilib>:"Mean.vi"("X"=w267) -> ("mean"=→"Mean Voltage":dbl)  [unwired: 1 out]
      n99 = Bundle By Name("t0"=w259, "dt"=w279, "Y"=w267) -> (w264:waveform(dbl))  [unwired: 1 in]
      "Avg Voltage" <- w264
      n100 = Bundle By Name("t0"=w259, "dt"=w279, "Y"=w268) -> (w265:waveform(dbl))  [unwired: 1 in]
      "Avg Current" <- w265
      n101 = call-poly <vilib>:"Get Waveform Time Array.vi"("waveform in"=w264) -> ("X array"=w269:timestamp[])  [unwired: 9 in, 1 out]
      n102 = To Double Precision Float(number=w269) -> (double precision float=w274:dbl[])
      n103 = call-poly <vilib>:"FFT Spectrum (Mag-Phase).vi"("window"=w286, "time signal"=w265) -> ("magnitude"=w262:cluster{"f0":dbl, "df":dbl, "magnitude":dbl[]})  [unwired: 5 in, 4 out]
      "Avg Current FFT" <- w262
      n104 = call-poly <vilib>:"FFT Spectrum (Mag-Phase).vi"("window"=w286, "time signal"=w264) -> ("magnitude"=w261:cluster{"f0":dbl, "df":dbl, "magnitude":dbl[]})  [unwired: 5 in, 4 out]
      "Avg Voltage FFT" <- w261
      n105 = Build Array(w274, w268, w267) -> (w273:dbl[][])
      n106 = Transpose 2D Array(2D array=w273) -> (transposed array=w272:dbl[][])
      "Output Data Array" <- w272
      n107 = case shown="True" "Write Time Data" {
        tunnel: w272 -> [_ w306]
        tunnel: w271 -> [_ w305]
        frame False {
        }
        frame True {
          # "Write File"
          n108 = call-poly <vilib>:"Write To Spreadsheet File.vi"("format (%.3f)"="%.10f", "append to file? (new file:F)"=TRUE, "2D data"=w306, "file path (dialog if empty)"=w305) -> ()  [unwired: 4 in, 1 out]
        }
      }
      n109 = Build Array(w262, w261) -> (→"Avg Data (FFT)":cluster{"f0":dbl, "df":dbl, "magnitude":dbl[]}[])
      n110 = Build Array(w265, w264) -> (→"Avg Data":waveform(dbl)[])
    }
  }
  n111 = Or(x=FALSE, y=w22) -> (x .or. y?=→"Measurement Complete":bool)
